vi "CC Script GUI.vi"(10 "Standalone":bool=TRUE, 11 "Cmd Qs":T1) -> ()   [LabVIEW 2024]
uses:
  Subsystems/SS cluster Command Queues.ctl
  Subsystems/SS typedef Cmd Queue Reference.ctl
  Subsystems/SS typedef cluster Instrument Command Queue Data.ctl
  CC cluster Script Panel Defaults.ctl
  typedefs/CC Script Step.ctl
  typedefs/CC enum Script Action.ctl
  typedefs/CC cluster Exposure.ctl
  Detector/Detector Class/Detector enum Detector Integration Mode.ctl
  typedefs/CC cluster Object.ctl
  typedefs/CC cluster sidereal rate.ctl
  typedefs/CC cluster RA and DEC.ctl
  typedefs/cc cluster muRA muDEC.ctl
  Telescope/CC cluster Telescope Offsets.ctl
  Telescope/Telescope cluster Equinox.ctl
  Telescope/Telescope cluster Parallax.ctl
  Telescope/Telescope cluster Rotator.ctl
  Telescope/Telesope ring Frame.ctl
  typedefs/CC cluster Acquire Parameters.ctl
  Subsystems/SS cluster Script Status Queue.ctl
  typedefs/CC cluster Random Dithering.ctl
  typedefs/CC Dithering.ctl
  typedefs/CC cluster Offset Dithering.ctl
  typedefs/CC Dithering Offsets.ctl
  typedefs/CC cluster Observation Record.ctl
  Subsystems/SS cluster New Image Data.ctl
  Subsystems/SS cluster Data Queue type.ctl
  typedefs/CC cluster Observation.ctl
  Observation Queue/CC enum Observation Status.ctl
  typedefs/CC cluster Observation Dither Options.ctl
  typedefs/CC enum Dither Selection.ctl
  hk-channel-class/hk-channel-class/HK Item/HK Item.lvclass
  typedefs/CC cluster Script.ctl
  typedefs/CC cluster Script Status Data.ctl
  typedefs/CC cluster Pause Parameters.ctl
  Filter Wheel/FW cmd Q Move Parameters.ctl
  Logging/CC enum Current Values Action.ctl
  Focus/Focus cluster MoveFocus Command Parameters.ctl
  typedefs/CC cluster Outlet Control.ctl
  CC Rd Wr Script Action.ctl
  e34a80dd-ae96-40f3-85ec-da568b1fc0c6.vi
  a150fa46-afdd-46f6-953a-6d695ab3cc3f.vi
  fb980131-14b8-4ba4-a5ba-d8795c8df878.vi
  73e8f019-b90d-454d-a375-f578a22e9470.vi
  6180e3d0-9506-4a5f-afbf-da5a1e2ce68c.vi
  79eba822-2b6b-4a1a-8f0f-f154aabb2b36.vi
  hk-channel-class/hk-channel-class/HK Table/HK Table.lvclass
  <vilib>/Utility/Data Type/NI_Data Type.lvlib
panel:
  in  "Script Path":path
  in  "Pause Button":bool
  out "Running":bool
  in  "Close":bool
  in  "Stop Script":bool
  in  "New Script":bool
  in  "Edit Script":bool
  in  "Run Script":bool
  in  "Script":string(combo)
  in  "Script":i32(listbox)
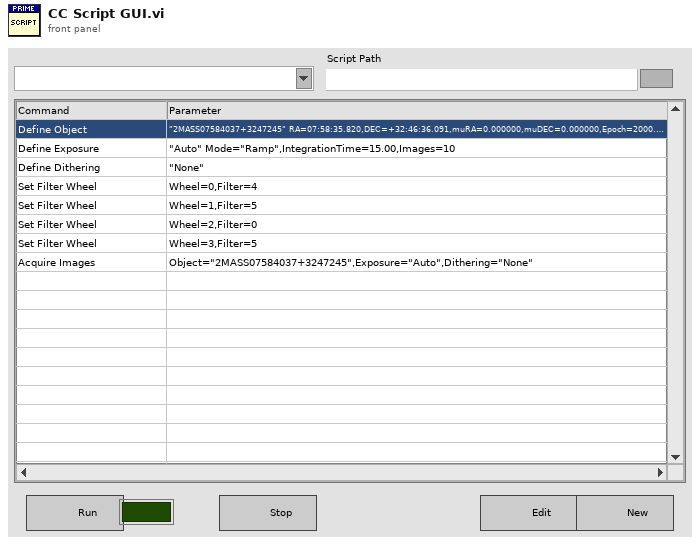
[diagram p1: front panel]
types:
  T1 = typedef "SS cluster Command Queues.ctl" = cluster{"Telescope Q":T2, "Filter Wheel Q":T2, "Script Q":T2, "CryoServer Q":T2, "Detector Q":T2, "Focus Q":T2, "Temp Ctl 1":T2, "Temp Ctl 2":T2, "Temp Ctl 3":T2, "CryoCooler Q":T2, "Pressure Q":T2}
  T2 = typedef "SS typedef Cmd Queue Reference.ctl" = refnum<queue>
  T3 = typedef "CC cluster Telescope Offsets.ctl" = cluster{"xi":dbl, "eta":dbl, "Offset Type":enum16{"SIMPLE", "TPLANE", "PA"}}
  T4 = typedef "CC cluster Script Panel Defaults.ctl" = cluster{"Script Name":string, "Script Path":path}
  T5 = typedef "CC Script Step.ctl" = cluster{"Action":T6, "Data":variant}
  T6 = typedef "CC enum Script Action.ctl" = enum16{"Noop", "Define Object", "Define Exposure", "Define Dithering", "Acquire Images", "Set Filter Wheel", "Telescope Home", "Telescope Move", "Telescope RA DEC", "Focus Move Relative", "Focus Move Absolute", "Focus Set Home", "Macro", "Pause", "Ask User", "Define Random Dither", "CmdLine", "Outlet"}
  T7 = typedef "CC cluster Exposure.ctl" = cluster{"Mode":T8, "Integration Time":dbl, "Name":string, "Images":i32}
  T8 = typedef "Detector enum Detector Integration Mode.ctl" = enum16{"Ramp", "CDS", "FOWLER2", "FOWLER4", "FOWLER8", "FOWLER16", "Raw"}
  T9 = typedef "CC cluster Object.ctl" = cluster{"Object":cluster{"Name":string}, "Sidereal Rate":T10, "RA and DEC":T11, "Proper Motion":T12, "Offsets":T3, "Equinox":T13, "Parallax":T14, "Rotator":T15, "Frame":T16, "Frac Rate":dbl, "Wavelength":dbl}
  T10 = typedef "CC cluster sidereal rate.ctl" = cluster{"dRA":dbl, "dDEC":dbl}
  T11 = typedef "CC cluster RA and DEC.ctl" = cluster{"RA":dbl, "DEC":dbl}
  T12 = typedef "cc cluster muRA muDEC.ctl" = cluster{"muRA":dbl, "muDEC":dbl, "Epoch":dbl}
  T13 = typedef "Telescope cluster Equinox.ctl" = cluster{"Equinox Year":i32, "Equinox Prefix":string}
  T14 = typedef "Telescope cluster Parallax.ctl" = cluster{"Parallax":dbl, "rv kps":dbl}
  T15 = typedef "Telescope cluster Rotator.ctl" = cluster{"Frame":enum16{"Target", "Fixed"}, "PA":dbl}
  T16 = typedef "Telesope ring Frame.ctl" = enum16{"FK4", "FK5", "APPT", "GAPPT", "AZEL"}
  T17 = typedef "CC cluster Acquire Parameters.ctl" = cluster{"Object":string, "Exposure":string, "Dithering":string}
  T18 = typedef "CC cluster Random Dithering.ctl" = cluster{"Count":i32, "Radius":dbl, "Name":string}
  T19 = typedef "CC Dithering.ctl" = cluster{"Name":string, "Dithering Offsets":T20}
  T20 = typedef "CC cluster Offset Dithering.ctl" = cluster{"Offsets":T21[]}
  T21 = typedef "CC Dithering Offsets.ctl" = cluster{"DEC":dbl, "RA":dbl}
  T22 = typedef "CC cluster Observation Record.ctl" = cluster{"Start Time":timestamp, "Script":string, "Object":string, "Detector Settings":string, "Dithering Type":string, "Filter":string, "Images":i32}
  T23 = typedef "SS cluster New Image Data.ctl" = cluster{"Frame number":i32, "Detector #":u16, "FITS file":path, "File size":i64, "Image Type":string}
  T24 = typedef "CC cluster Observation.ctl" = cluster{"Priority":i32, "ID":string, "Observer":string, "Obj Name":string, "Obj Type":string, "RA and DEC String":cluster{"RA":string, "DEC":string}, "Filters":string[], "Integration Time":dbl, "Observation Status":T25, "Offsets":T3, "Images":i32, "Dither Options":T26, "Comment 1":string, "Comment 2":string, "Rotator":T15}
  T25 = typedef "CC enum Observation Status.ctl" = enum16{"Ready", "Running", "Done", "Error"}
  T26 = typedef "CC cluster Observation Dither Options.ctl" = cluster{"Dither":T27, "Dither Radius":dbl, "Dither Points":i32, "Dither Phase":dbl, "B Offset":T11}
  T27 = typedef "CC enum Dither Selection.ctl" = enum16{"None", "Circle", "Random", "ABBA", "OnOff"}
  T28 = cluster{"state":refnum<user-event>, "Script Settings":T4, "Script":T5[], "Cmd Qs":T1, "Parameters":variant, "step":i32, "Script Running":bool, "timer":timestamp, "Script State":string, "Exposure":T7, "Object Map":map{string, T9}, "Acq Settings":T17, "target":T9, "Exp Map":map{string, T7}, "Script Status Q":refnum<queue>, "Images Received":bool, "script edit ref":refnum<vi>, "Run Script":T5[], "Dither":cluster{"Dither Type":bool, "Random Dither":T18, "Offset Dithering":T19, "index":i32}, "Obs List":T22[], "Obs":T22, "images":T23[], "Data Q":refnum<queue>, "Total Images":i32, "paused":bool, "Target RA and DEC":T11, "Image idx":i32, "Observation":T24, "Channel List":refnum<class "HK Item.lvclass">[], "Dither Map":map{string, cluster{"Dither Type":bool, "Random Dither":T18, "Offset Dithering":T19, "index":i32}}, "move start":timestamp, "at slit?":bool, "obj name":string}
  T29 = enum8{"Enabled", "Disabled", "Disabled and Grayed Out"}
  T30 = typedef "SS typedef cluster Instrument Command Queue Data.ctl" = cluster{"Cmd":string, "Parameters":variant}
  T31 = typedef "SS cluster Data Queue type.ctl" = cluster{"Source":string, "Type":string, "Data":variant}
  T32 = typedef "SS cluster Script Status Queue.ctl" = cluster{"Msg":string, "Data":variant}
  T33 = typedef "CC cluster Script.ctl" = cluster{"Name":string, "Script":T5[]}
  T34 = cluster{"Dither Type":bool, "Random Dither":T18, "Offset Dithering":T19, "index":i32}
  T35 = typedef "CC cluster Script Status Data.ctl" = cluster{"Time":timestamp, "Running":bool, "Step":i32, "Script Name":string, "Step Name":string}
  T36 = typedef "CC cluster Pause Parameters.ctl" = cluster{"Time (s)":dbl}
  T37 = typedef "CC enum Current Values Action.ctl" = enum16{"Init", "Write Item", "Write Array", "Read Item", "Read Array", "Read All", "Add Channels", "New File", "Add Message", "Get Current Values", "Close"}
  T38 = typedef "FW cmd Q Move Parameters.ctl" = cluster{"Wheel ID":i32, "Position":i32}
  T39 = typedef "Focus cluster MoveFocus Command Parameters.ctl" = cluster{"Motor":i32, "Position":i32}
  T40 = typedef "CC cluster Outlet Control.ctl" = cluster{"Outlet Idx":i32, "State":bool}
  T41 = typedef "CC Rd Wr Script Action.ctl" = enum16{"Read", "Write", "List", "Delete"}
  T42 = map{string, cluster{"Dither Type":bool, "Random Dither":T18, "Offset Dithering":T19, "index":i32}}
  T43 = typedef "CC cluster Dithering.ctl" = cluster{"Dither Type":bool, "Random Dither":T18, "Offset Dithering":T19, "index":i32}
  T44 = typedef "LVPoint32TypeDef.ctl" = cluster{"Horizontal":i32, "Vertical":i32}
  T45 = typedef "LVRowAndColumnTypeDef.ctl" = cluster{"Row":i32, "Column":i32}
  T46 = enum32{"Invalid", "Standard", "Closed", "Hidden", "Minimized", "Maximized"}
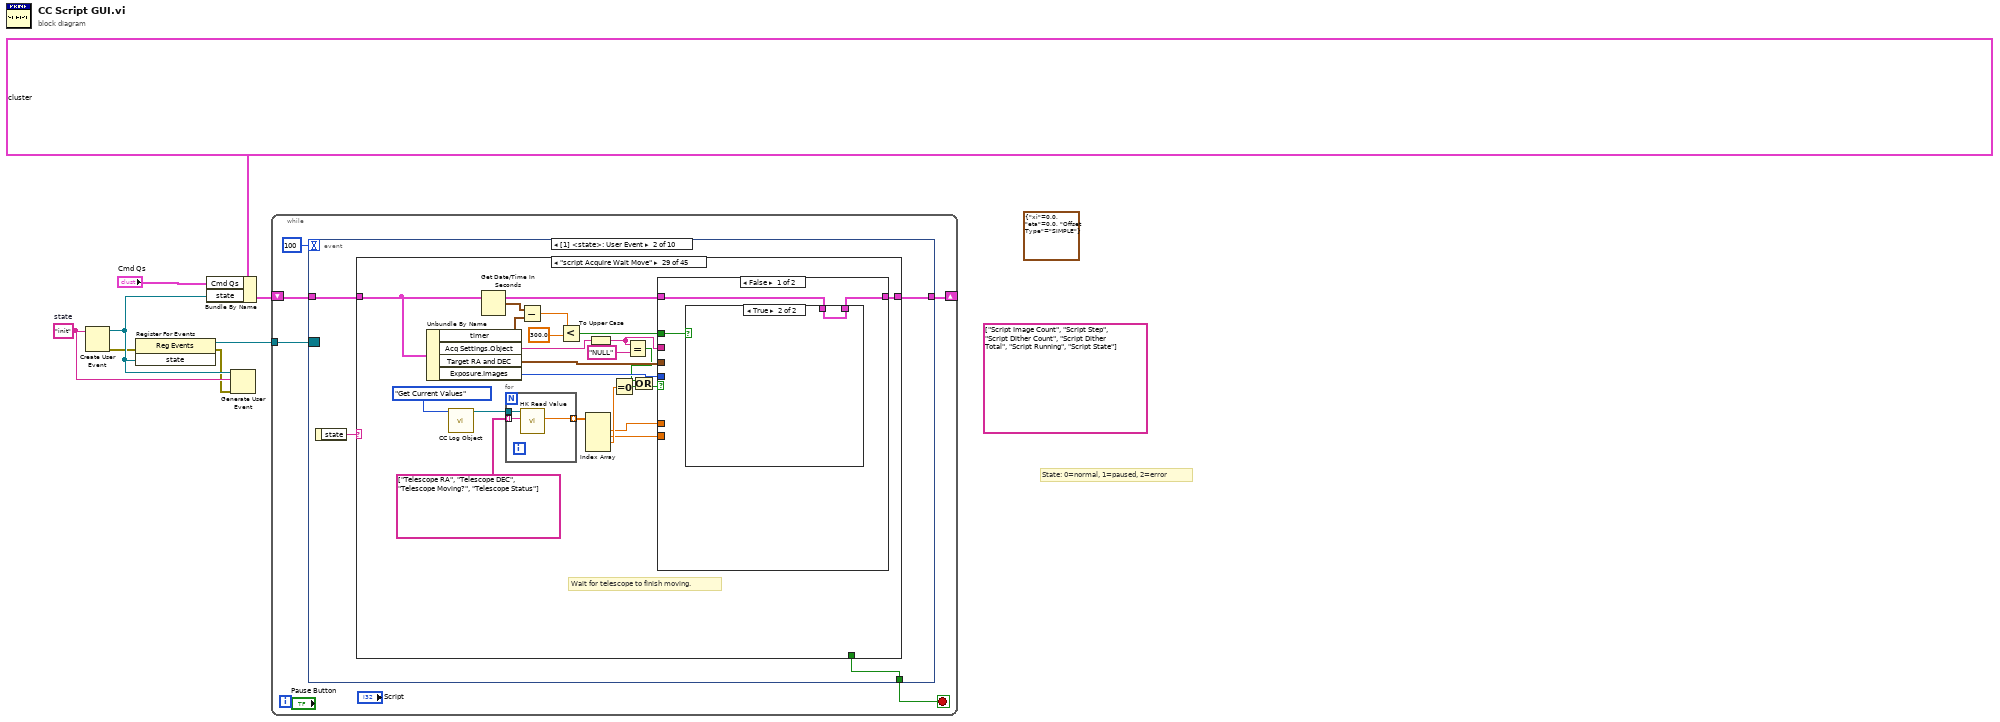
[diagram p0: block diagram]
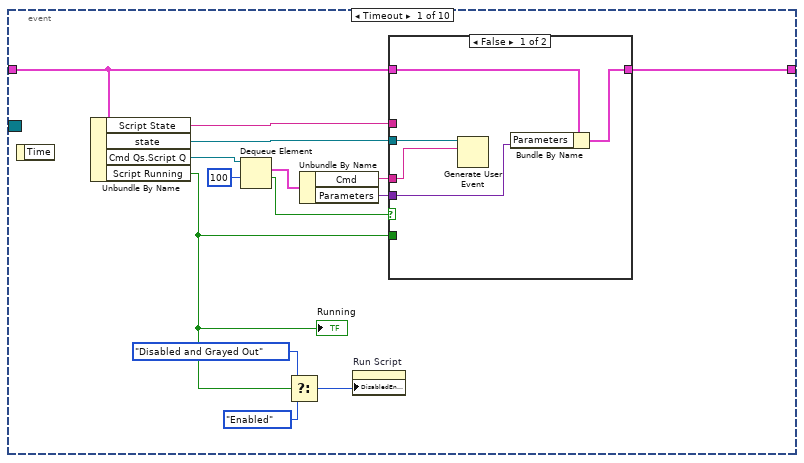
[diagram p2: hidden frame]
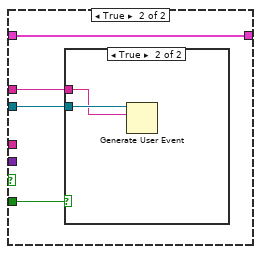
[diagram p3: hidden frame]
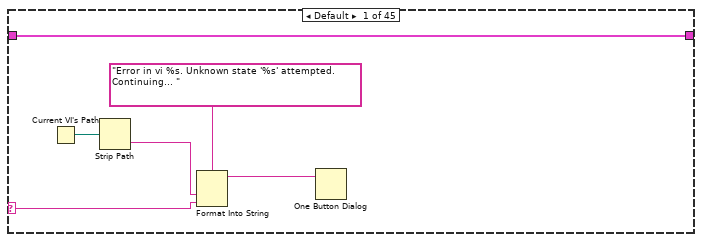
[diagram p5: hidden frame]
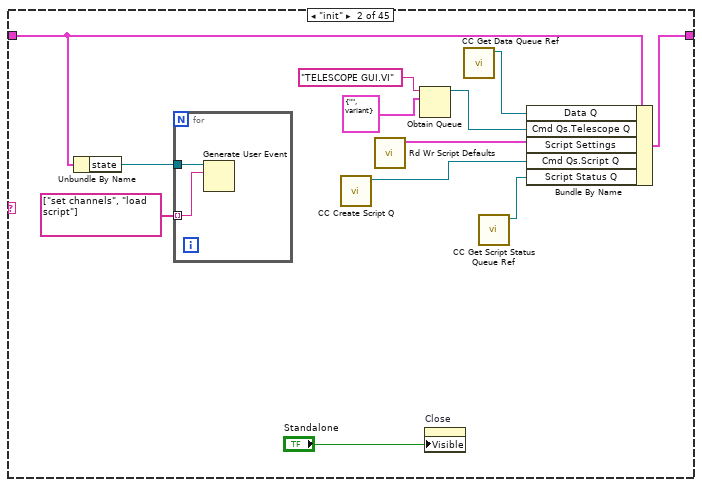
[diagram p6: hidden frame]
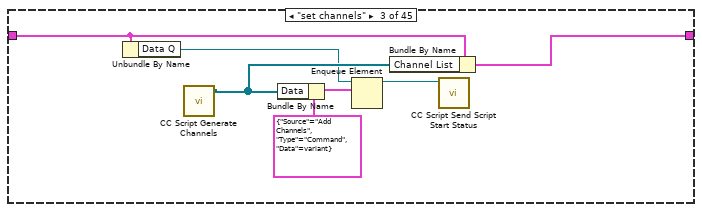
[diagram p7: hidden frame]
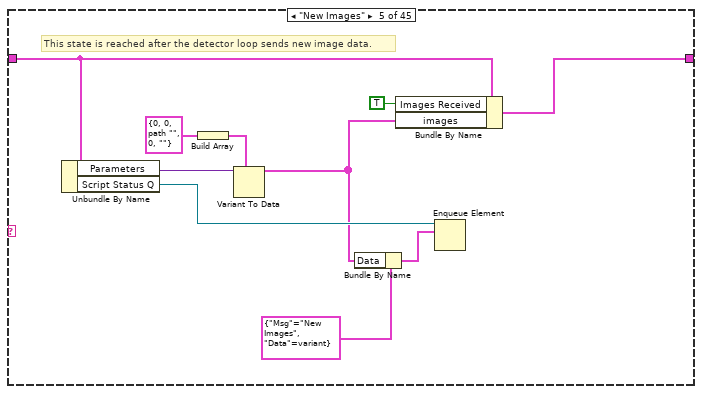
[diagram p9: hidden frame]
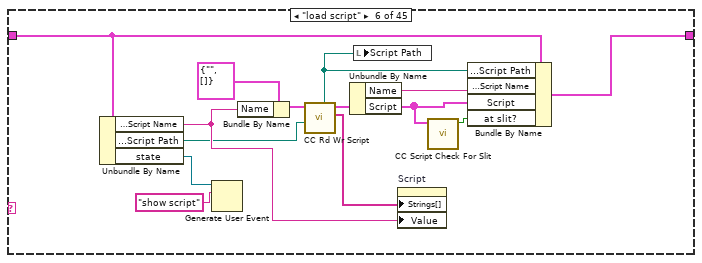
[diagram p10: hidden frame]
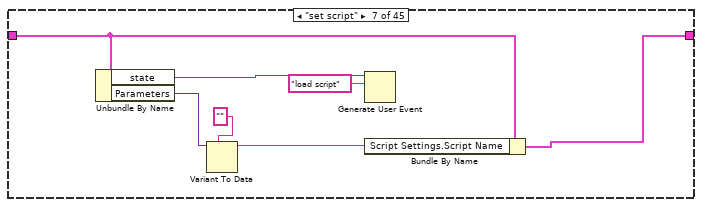
[diagram p11: hidden frame]
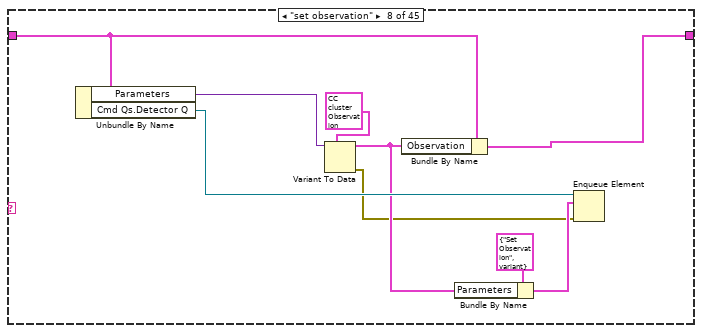
[diagram p12: hidden frame]
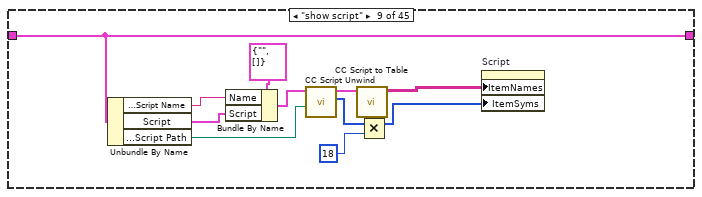
[diagram p13: hidden frame]
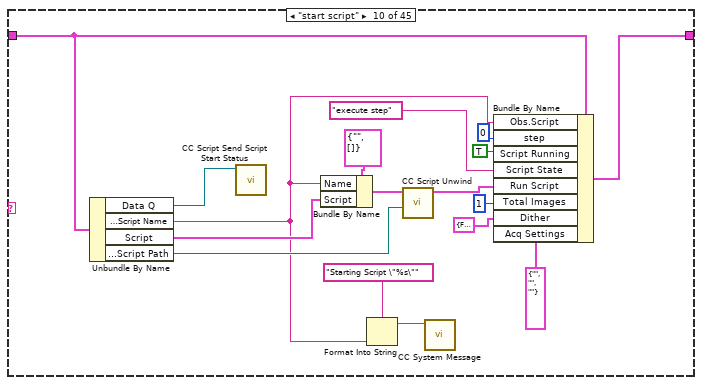
[diagram p14: hidden frame]
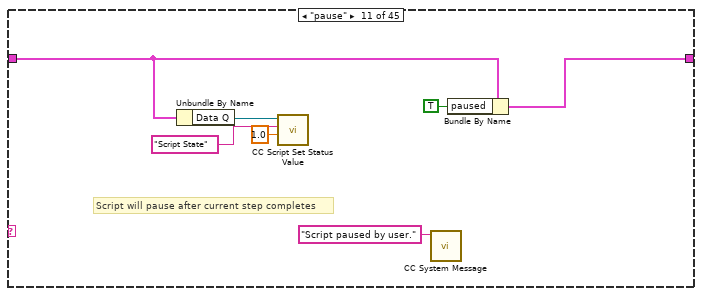
[diagram p15: hidden frame]
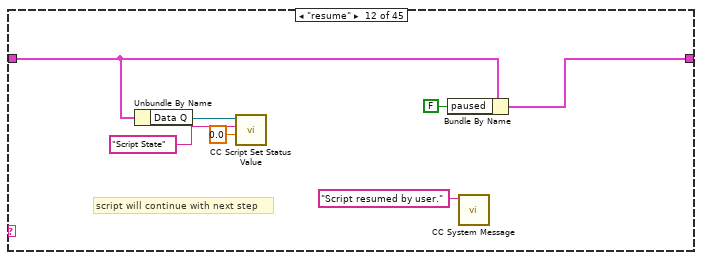
[diagram p16: hidden frame]
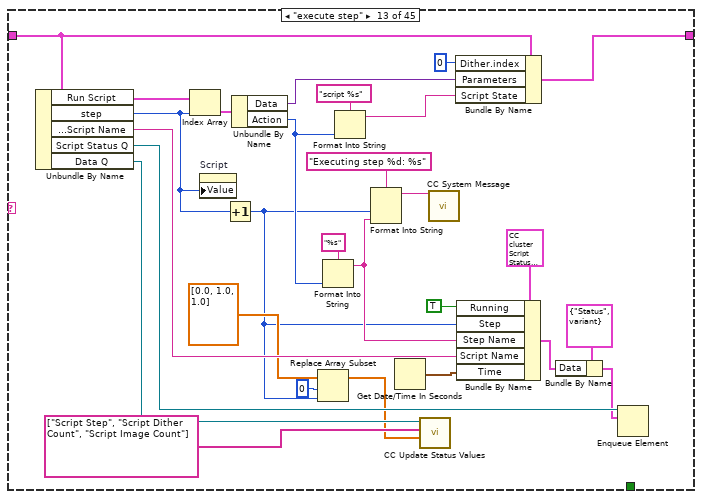
[diagram p17: hidden frame]
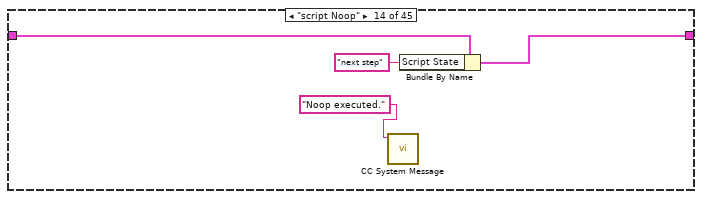
[diagram p18: hidden frame]
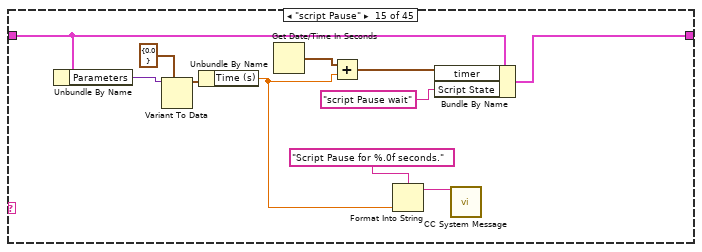
[diagram p19: hidden frame]
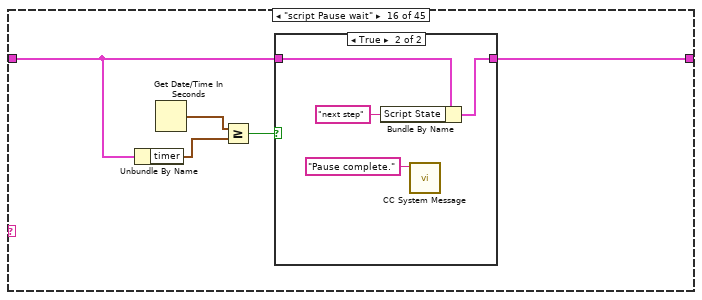
[diagram p20: hidden frame]
diagram:
  (unwired) T3 {"xi"=0.0, "eta"=0.0, "Offset Type"=enum."SIMPLE"} ("Offsets")
  (unwired) string[] ["Script Image Count", "Script Step", "Script Dither Count", "Script Dither Total", "Script Running", "Script State"]
  w4 = "init"  # state
  # "State: 0=normal, 1=paused, 2=error"
  n1 = Create User Event(user event datatype=w4) -> (user event=w6:refnum<user-event>, error out=w2:errorcluster)  [unwired: 1 in]
  n2 = register-events(error in=w2, w6) -> (reference out=w5:refnum<event-registration>, error out=w3:errorcluster)  [unwired: 1 in]
  n3 = Bundle By Name(cluster=T28 {"state"=refnum, "Script Settings"={"Script Name"="", "Script Path"=path ""}, "Script"=[], "Cmd Qs"={"Telescope Q"=refnum, "Filter Wheel Q"=refnum, "Script Q"=refnum, "CryoServer Q"=refnum, "Detector Q"=refnum, "Focus Q"=refnum, "Temp Ctl 1"=refnum, "Temp Ctl 2"=refnum, "Temp Ctl 3"=refnum, "CryoCooler Q"=refnum, "Pressure Q"=refnum}, "Parameters"=variant, "step"=0, "Script Running"=FALSE, "timer"=timestamp(0 s since 1904-01-01), "Script State"="", "Exposure"={"Mode"=enum."CDS", "Integration Time"=1.0, "Name"="", "Images"=1}, "Object Map"={}, "Acq Settings"={"Object"="", "Exposure"="", "Dithering"=""}, "target"={"Object"={"Name"=""}, "Sidereal Rate"={"dRA"=0.0, "dDEC"=0.0}, "RA and DEC"={"RA"=0.0, "DEC"=0.0}, "Proper Motion"={"muRA"=0.0, "muDEC"=0.0, "Epoch"=0.0}, "Offsets"={"xi"=0.0, "eta"=0.0, "Offset Type"=enum."SIMPLE"}, "Equinox"={"Equinox Year"=2000, "Equinox Prefix"="J"}, "Parallax"={"Parallax"=0.0, "rv kps"=0.0}, "Rotator"={"Frame"=enum."Target", "PA"=0.0}, "Frame"=enum."FK5", "Frac Rate"=1.0, "Wavelength"=0.5}, "Exp Map"={}, "Script Status Q"=refnum, "Images Received"=FALSE, "script edit ref"=refnum, "Run Script"=[], "Dither"={"Dither Type"=FALSE, "Random Dither"={"Count"=1, "Radius"=1.0, "Name"=""}, "Offset Dithering"={"Name"="", "Dithering Offsets"={"Offsets"=[]}}, "index"=0}, "Obs List"=[], "Obs"={"Start Time"=timestamp(0 s since 1904-01-01), "Script"="", "Object"="", "Detector Settings"="", "Dithering Type"="", "Filter"="", "Images"=0}, "images"=[], "Data Q"=refnum, "Total Images"=0, "paused"=FALSE, "Target RA and DEC"={"RA"=0.0, "DEC"=0.0}, "Image idx"=0, "Observation"={"Priority"=0, "ID"="", "Observer"="", "Obj Name"="", "Obj Type"="", "RA and DEC String"={"RA"="HH:MM:SS.nnn", "DEC"="DEG:arcmin:arcsec.nn"}, "Filters"=[], "Integration Time"=0.0, "Observation Status"=enum."Ready", "Offsets"={"xi"=0.0, "eta"=0.0, "Offset Type"=enum."SIMPLE"}, "Images"=0, "Dither Options"={"Dither"=enum."None", "Dither Radius"=0.0, "Dither Points"=0, "Dither Phase"=0.0, "B Offset"={"RA"=0.0, "DEC"=0.0}}, "Comment 1"="", "Comment 2"="", "Rotator"={"Frame"=enum."Target", "PA"=0.0}}, "Channel List"=[], "Dither Map"={}, "move start"=timestamp(0 s since 1904-01-01), "at slit?"=FALSE, "obj name"=""}, "Cmd Qs"="Cmd Qs", "state"=w6) -> (w7:T28)
  n4 = Generate User Event(user event=w6, event data cluster=w4, error in=w3) -> ()  [unwired: 1 in, 2 out]
  n5 = while {
    tunnel: w5 -> [w13]
    shift-right: [w11] -> _
    shift-left: w7 -> [w12]
    stop <- w10 stop-if-true
    n6 = event shown="[1] <state>: User Event" {
      selector: w13 -> [_ _ _ _ _ _ _ _ _ _]
      dyn-events: _ -> [_ _ _ _ _ _ _ _ _ _]
      timeout: 100 -> [_ _ _ _ _ _ _ _ _ _]
      tunnel: w12 -> [w21 w41 w755 w758 w773 w815 w820 w842 w845 w848]
      tunnel: [w19 w40 w752 w758 w772 w816 w821 w842 w845 w848] -> w11
      tunnel: [_ w39 _ _ _ _ _ _ _ _] -> w10
      event Timeout {
        n7 = event-data() -> ()  [unwired: 1 in, 1 out]
        n8 = Unbundle By Name(w21) -> ("Script State"=w18:string, "state"=w22:refnum<user-event>, "Cmd Qs.Script Q"=w27:T2, "Script Running"=w17:bool)
        "Running" <- w17
        n9 = Dequeue Element(queue=w27, timeout in ms (-1)=100) -> (element=w25:T30, timed out?=w24:bool)  [unwired: 1 in, 2 out]
        n10 = Select(t=T29."Disabled and Grayed Out" ("Disabled"), s=w17, f=T29."Enabled" ("Disabled")) -> (s? t:f=w14:T29)
        n11 = Unbundle By Name(w25) -> ("Cmd"=w23:string, "Parameters"=w20:variant)
        n12 = property on="Run Script" class="Bool"("DisabledEnum"=w14) -> ()  [unwired: 2 in, 2 out]
        n13 = case shown="False" w24 {
          tunnel: w23 -> [w31 _]
          tunnel: w22 -> [w32 w34]
          tunnel: w21 -> [w30 w36]
          tunnel: w20 -> [w29 _]
          tunnel: [w28 w36] -> w19
          tunnel: w17 -> [_ w35]
          tunnel: w18 -> [_ w33]
          frame False {
            n14 = Generate User Event(user event=w32, event data cluster=w31) -> ()  [unwired: 2 in, 2 out]
            n15 = Bundle By Name(cluster=w30, "Parameters"=w29) -> (w28:T28)
          }
          frame True {
            n16 = case shown="True" w35 {
              tunnel: w34 -> [_ w38]
              tunnel: w33 -> [_ w37]
              frame False {
              }
              frame True {
                n17 = Generate User Event(user event=w38, event data cluster=w37) -> ()  [unwired: 2 in, 2 out]
              }
            }
          }
        }
      }
      event User Event {
        n18 = event-data() -> ("state"=w42:string)  [unwired: 1 in]
        n19 = case shown="\"script Acquire Wait Move\"" w42 {
          selector: w42 -> [w47 _ _ _ _ _ _ _ _ _ _ _ _ _ _ _ _ _ _ _ _ _ w339 _ _ _ w388 _ _ _ w515 _ _ _ _ _ _ _ _ _ _ _ _ _ _]
          tunnel: w41 -> [w43 w58 w65 w70 w75 w86 w96 w108 w121 w137 w140 w150 w172 w181 w186 w197 w210 w242 w261 w281 w301 w332 w341 w364 w374 w385 w390 w426 w450 w498 w512 w527 w552 w576 w589 w612 w626 w650 w651 w666 w693 w721 w729 w740 w748]
          tunnel: [w43 w59 w66 w70 w76 w87 w97 w109 w121 w138 w144 w151 w173 w182 w187 w196 w213 w243 w264 w284 w304 w306 w342 w366 w376 w387 w391 w427 w453 w499 w513 w529 w550 w577 w590 w613 w627 w650 w652 w667 w691 w722 w730 w744 w748] -> w40
          tunnel: [_ _ _ _ _ _ _ _ _ _ _ _ _ _ _ _ _ _ _ _ _ _ _ _ _ _ _ _ _ _ _ _ _ _ _ _ _ _ _ _ _ _ _ _ TRUE] -> w39
          frame Default {
            n20 = Current VI's Path() -> (path=w46:path)
            n21 = Strip Path(path=w46) -> (name=w45:string)  [unwired: 1 out]
            n22 = Format Into String(format string="Error in vi %s. Unknown state '%s' attempted. Continuing... ", w45, w47) -> (resulting string=w44:string)  [unwired: 2 in, 1 out]
            n23 = One Button Dialog(message=w44) -> ()  [unwired: 1 in, 1 out]
          }
          frame "init" {
            n24 = Unbundle By Name(w58) -> ("state"=w57:refnum<user-event>)
            n25 = for {
              tunnel: w57 -> [w62]
              tunnel: string[] ["set channels", "load script"] -> [w61] mode=indexing
              n26 = Generate User Event(user event=w62, event data cluster=w61) -> ()  [unwired: 2 in, 2 out]
            }
            n27 = call "CC Create Script Q.vi"() -> ("Script Q"=w49:refnum<queue>)  [unwired: 10 in, 1 out]
            n28 = call "Rd Wr Script Defaults.vi"() -> ("Script Settings"=w60:T4)  [unwired: 10 in, 1 out]
            n29 = Obtain Queue(name (unnamed)="TELESCOPE GUI.VI", element data type=T30 {"Cmd"="", "Parameters"=variant}) -> (queue out=w52:refnum<queue>)  [unwired: 3 in, 2 out]
            n30 = property on="Close" class="Bool"("Visible"="Standalone") -> ()  [unwired: 2 in, 2 out]
            n31 = call "CC Get Data Queue Ref.vi"() -> ("Data Q"=w50:refnum<queue>)  [unwired: 10 in, 1 out]
            n32 = call "CC Get Script Status Queue Ref.vi"() -> ("Script Status Q"=w55:refnum<queue>)  [unwired: 10 in, 1 out]
            n33 = Bundle By Name(cluster=w58, "Data Q"=w50, "Cmd Qs.Telescope Q"=w52, "Script Settings"=w60, "Cmd Qs.Script Q"=w49, "Script Status Q"=w55) -> (w59:T28)
          }
          frame "set channels" {
            n34 = Unbundle By Name(w65) -> ("Data Q"=w64:refnum<queue>)
            n35 = call "CC Script Generate Channels.vi"() -> ("Channel List"=w67:refnum<class "HK Item.lvclass">[])  [unwired: 9 in, 2 out]
            n36 = Bundle By Name(cluster=T31 {"Source"="Add Channels", "Type"="Command", "Data"=variant} ("element"), "Data"=w67) -> (w69:T31)
            n37 = Enqueue Element(queue=w64, element=w69) -> (queue out=w63:refnum<queue>)  [unwired: 2 in, 2 out]
            n38 = Bundle By Name(cluster=w65, "Channel List"=w67) -> (w66:T28)
            n39 = call "CC Script Send Script Start Status.vi"("Data Q"=w63) -> ()  [unwired: 10 in, 1 out]
          }
          frame "idle" {
          }
          frame "New Images" {
            # "This state is reached after the detector loop sends new image data."
            n40 = Unbundle By Name(w75) -> ("Parameters"=w79:variant, "Script Status Q"=w74:refnum<queue>)
            n41 = Build Array(T23 {"Frame number"=0, "Detector #"=0, "FITS file"=path "", "File size"=0, "Image Type"=""} ("New Image")) -> (w78:T23[])
            n42 = Variant To Data(type=w78, Variant=w79) -> (data=w71:T23[])  [unwired: 1 in, 1 out]
            n43 = Bundle By Name(cluster=T32 {"Msg"="New Images", "Data"=variant} ("element"), "Data"=w71) -> (w72:T32)
            n44 = Bundle By Name(cluster=w75, "Images Received"=TRUE, "images"=w71) -> (w76:T28)
            n45 = Enqueue Element(queue=w74, element=w72) -> ()  [unwired: 2 in, 3 out]
          }
          frame "load script" {
            n46 = Unbundle By Name(w86) -> ("Script Settings.Script Name"=w85:string, "Script Settings.Script Path"=w84:path, "state"=w89:refnum<user-event>)
            n47 = Generate User Event(user event=w89, event data cluster="show script" ("event data")) -> ()  [unwired: 2 in, 2 out]
            n48 = Bundle By Name(cluster=T33 {"Name"="", "Script"=[]} ("Script"), "Name"=w85) -> (w94:T33)
            n49 = call "CC Rd Wr Script.vi"("Script Path"=w84, "Script"=w94) -> ("Script List"=w92:string[], "Script"=w93:T33, "Script Path"=w83:path)  [unwired: 4 in, 3 out]
            n50 = Unbundle By Name(w93) -> ("Name"=w88:string, "Script"=w82:T5[])
            n51 = local write "Script Path"(w83) -> ()
            n52 = property on="Script" class="CmbBox"("Strings[]"=w92, "Value"=w85) -> ()  [unwired: 2 in, 2 out]
            n53 = call "CC Script Check For Slit.vi"("Script"=w82) -> ("At Slit?"=w81:bool)  [unwired: 9 in, 1 out]
            n54 = Bundle By Name(cluster=w86, "Script Settings.Script Path"=w83, "Script Settings.Script Name"=w88, "Script"=w82, "at slit?"=w81) -> (w87:T28)
          }
          frame "set script" {
            n55 = Unbundle By Name(w96) -> ("state"=w99:refnum<user-event>, "Parameters"=w101:variant)
            n56 = Variant To Data(type="", Variant=w101) -> (data=w98:string)  [unwired: 1 in, 1 out]
            n57 = Generate User Event(user event=w99, event data cluster="load script" ("event data")) -> ()  [unwired: 2 in, 2 out]
            n58 = Bundle By Name(cluster=w96, "Script Settings.Script Name"=w98) -> (w97:T28)
          }
          frame "set observation" {
            n59 = Unbundle By Name(w108) -> ("Parameters"=w110:variant, "Cmd Qs.Detector Q"=w106:T2)
            n60 = Variant To Data(type=T24 {"Priority"=0, "ID"="", "Observer"="", "Obj Name"="", "Obj Type"="", "RA and DEC String"={"RA"="HH:MM:SS.nnn", "DEC"="DEG:arcmin:arcsec.nn"}, "Filters"=[], "Integration Time"=0.0, "Observation Status"=enum."Error", "Offsets"={"xi"=0.0, "eta"=0.0, "Offset Type"=enum."SIMPLE"}, "Images"=0, "Dither Options"={"Dither"=enum."None", "Dither Radius"=0.0, "Dither Points"=0, "Dither Phase"=0.0, "B Offset"={"RA"=0.0, "DEC"=0.0}}, "Comment 1"="", "Comment 2"="", "Rotator"={"Frame"=enum."Target", "PA"=0.0}} ("element"), Variant=w110) -> (data=w103:T24, error out=w102:errorcluster)  [unwired: 1 in]
            n61 = Bundle By Name(cluster=w108, "Observation"=w103) -> (w109:T28)
            n62 = Bundle By Name(cluster=T30 {"Cmd"="Set Observation", "Parameters"=variant} ("element"), "Parameters"=w103) -> (w104:T30)
            n63 = Enqueue Element(queue=w106, element=w104, error in (no error)=w102) -> ()  [unwired: 1 in, 3 out]
          }
          frame "show script" {
            n64 = Unbundle By Name(w121) -> ("Script Settings.Script Name"=w118:string, "Script"=w117:T5[], "Script Settings.Script Path"=w111:path)
            n65 = Bundle By Name(cluster=T33 {"Name"="", "Script"=[]} ("Script"), "Name"=w118, "Script"=w117) -> (w116:T33)
            n66 = call "CC Script Unwind.vi"("Script Path"=w111, "Script"=w116) -> ("Indent"=w114:i32[], "Unwound Script"=w115:T5[])  [unwired: 7 in, 1 out]
            n67 = call "CC Script to Table.vi"("Script"=w115) -> ("table"=w120:string[][])  [unwired: 9 in, 1 out]
            n68 = Multiply(x=w114, y=18) -> (x*y=w113:i32[])
            n69 = property on="Script" class="MCListbox (strict)"("ItemNames"=w120, "ItemSyms"=w113) -> ()  [unwired: 2 in, 2 out]
          }
          frame "start script" {
            n70 = Unbundle By Name(w137) -> ("Data Q"=w125:refnum<queue>, "Script Settings.Script Name"=w126:string, "Script"=w130:T5[], "Script Settings.Script Path"=w127:path)
            n71 = call "CC Script Send Script Start Status.vi"("Data Q"=w125) -> ()  [unwired: 10 in, 1 out]
            n72 = Bundle By Name(cluster=T33 {"Name"="", "Script"=[]} ("Script"), "Name"=w126, "Script"=w130) -> (w129:T33)
            n73 = Format Into String(format string="Starting Script \"%s\"" ("Message"), w126) -> (resulting string=w134:string)  [unwired: 2 in, 1 out]
            n74 = call "CC Script Unwind.vi"("Script Path"=w127, "Script"=w129) -> ("Unwound Script"=w128:T5[])  [unwired: 7 in, 2 out]
            n75 = call "CC System Message.vi"("Message"=w134) -> ()  [unwired: 10 in, 1 out]
            n76 = Bundle By Name(cluster=w137, "Obs.Script"=w126, "step"=0, "Script Running"=TRUE, "Script State"="execute step" ("event data"), "Run Script"=w128, "Total Images"=1 ("Image Count"), "Dither"=T34 {"Dither Type"=FALSE, "Random Dither"={"Count"=0, "Radius"=0.0, "Name"=""}, "Offset Dithering"={"Name"="", "Dithering Offsets"={"Offsets"=[]}}, "index"=0}, "Acq Settings"=T17 {"Object"="", "Exposure"="", "Dithering"=""}) -> (w138:T28)
          }
          frame "pause" {
            # "Script will pause after current step completes"
            n77 = Unbundle By Name(w140) -> ("Data Q"=w143:refnum<queue>)
            n78 = call "CC Script Set Status Value.vi"("Value"=1.0, "Ch Name"="Script State", "Data Q"=w143) -> ()  [unwired: 8 in, 1 out]
            n79 = call "CC System Message.vi"("Message"="Script paused by user.") -> ()  [unwired: 10 in, 1 out]
            n80 = Bundle By Name(cluster=w140, "paused"=TRUE) -> (w144:T28)
          }
          frame "resume" {
            # "script will continue with next step"
            n81 = Unbundle By Name(w150) -> ("Data Q"=w149:refnum<queue>)
            n82 = call "CC Script Set Status Value.vi"("Value"=0.0, "Ch Name"="Script State", "Data Q"=w149) -> ()  [unwired: 8 in, 1 out]
            n83 = Bundle By Name(cluster=w150, "paused"=FALSE) -> (w151:T28)
            n84 = call "CC System Message.vi"("Message"="Script resumed by user.") -> ()  [unwired: 10 in, 1 out]
          }
          frame "execute step" {
            n85 = Unbundle By Name(w172) -> ("Run Script"=w180:T5[], "step"=w176:i32, "Script Settings.Script Name"=w165:string, "Script Status Q"=w163:refnum<queue>, "Data Q"=w158:refnum<queue>)
            n86 = Index Array(array=w180, index=w176) -> (element=w179:T5)
            n87 = property on="Script" class="MCListbox (strict)"("Value"=w176) -> ()  [unwired: 2 in, 2 out]
            n88 = Increment(x=w176) -> (x+1=w154:i32)
            n89 = Unbundle By Name(w179) -> ("Data"=w171:variant, "Action"=w167:T6)
            n90 = Replace Array Subset(array=dbl[] [0.0, 1.0, 1.0] ("Values"), new element=w154, index=0) -> (w153:dbl[])
            n91 = Format Into String(format string="%s", w167) -> (resulting string=w166:string)  [unwired: 2 in, 1 out]
            n92 = Format Into String(format string="script %s", w167) -> (resulting string=w174:string)  [unwired: 2 in, 1 out]
            n93 = Format Into String(format string="Executing step %d: %s", w154, w166) -> (resulting string=w175:string)  [unwired: 2 in, 1 out]
            n94 = Get Date/Time In Seconds() -> (seconds since 1Jan1904=w164:timestamp)
            n95 = call "CC Update Status Values.vi"("Values"=w153, "names"=string[] ["Script Step", "Script Dither Count", "Script Image Count"], "Data Q"=w158) -> ()  [unwired: 8 in, 1 out]
            n96 = call "CC System Message.vi"("Message"=w175) -> ()  [unwired: 10 in, 1 out]
            n97 = Bundle By Name(cluster=w172, "Dither.index"=0, "Parameters"=w171, "Script State"=w174) -> (w173:T28)
            n98 = Bundle By Name(cluster=T35 {"Time"=timestamp(0 s since 1904-01-01), "Running"=FALSE, "Step"=0, "Script Name"="", "Step Name"=""}, "Running"=TRUE, "Step"=w154, "Step Name"=w166, "Script Name"=w165, "Time"=w164) -> (w161:T35)
            n99 = Bundle By Name(cluster=T32 {"Msg"="Status", "Data"=variant} ("element"), "Data"=w161) -> (w160:T32)
            n100 = Enqueue Element(queue=w163, element=w160) -> ()  [unwired: 2 in, 3 out]
          }
          frame "script Noop" {
            n101 = call "CC System Message.vi"("Message"="Noop executed." ("format string")) -> ()  [unwired: 10 in, 1 out]
            n102 = Bundle By Name(cluster=w181, "Script State"="next step" ("event data")) -> (w182:T28)
          }
          frame "script Pause" {
            n103 = Unbundle By Name(w186) -> ("Parameters"=w193:variant)
            n104 = Variant To Data(type=T36 {"Time (s)"=0.0} ("Pause Parameters"), Variant=w193) -> (data=w191:T36)  [unwired: 1 in, 1 out]
            n105 = Unbundle By Name(w191) -> ("Time (s)"=w189:dbl)
            n106 = Get Date/Time In Seconds() -> (seconds since 1Jan1904=w190:timestamp)
            n107 = Add(x=w190, y=w189) -> (x+y=w188:timestamp)
            n108 = Format Into String(format string="Script Pause for %.0f seconds.", w189) -> (resulting string=w194:string)  [unwired: 2 in, 1 out]
            n109 = Bundle By Name(cluster=w186, "timer"=w188, "Script State"="script Pause wait" ("event data")) -> (w187:T28)
            n110 = call "CC System Message.vi"("Message"=w194) -> ()  [unwired: 10 in, 1 out]
          }
          frame "script Pause wait" {
            n111 = Unbundle By Name(w197) -> ("timer"=w199:timestamp)
            n112 = Get Date/Time In Seconds() -> (seconds since 1Jan1904=w200:timestamp)
            n113 = Greater Or Equal?(x=w200, y=w199) -> (x >= y?=w198:bool)
            n114 = case shown="True" w198 {
              tunnel: w197 -> [w201 w205]
              tunnel: [w201 w203] -> w196
              frame False {
              }
              frame True {
                n115 = Bundle By Name(cluster=w205, "Script State"="next step") -> (w203:T28)
                n116 = call "CC System Message.vi"("Message"="Pause complete.") -> ()  [unwired: 10 in, 1 out]
              }
            }
          }
          frame "script Macro" {
            n117 = Unbundle By Name(w210) -> ("Parameters"=w211:variant)
            n118 = Variant To Data(type="", Variant=w211) -> (data=w207:string)  [unwired: 1 in, 1 out]
            n119 = Format Into String(format string="Executing Macro %s" ("Message"), w207) -> (resulting string=w206:string)  [unwired: 2 in, 1 out]
            n120 = Bundle By Name(cluster=w210, "Script State"="next step") -> (w213:T28)
            n121 = call "CC System Message.vi"("Message"=w206) -> ()  [unwired: 10 in, 1 out]
          }
          frame "script Define Object" {
            n122 = Unbundle By Name(w242) -> ("Parameters"=w241:variant, "Object Map"=w239:map{string, T9}, "at slit?"=w219:bool, "Cmd Qs.Telescope Q"=w230:T2)
            n123 = Variant To Data(type=T9 {"Object"={"Name"=""}, "Sidereal Rate"={"dRA"=0.0, "dDEC"=0.0}, "RA and DEC"={"RA"=0.0, "DEC"=0.0}, "Proper Motion"={"muRA"=0.0, "muDEC"=0.0, "Epoch"=0.0}, "Offsets"={"xi"=0.0, "eta"=0.0, "Offset Type"=enum."SIMPLE"}, "Equinox"={"Equinox Year"=2000, "Equinox Prefix"="J"}, "Parallax"={"Parallax"=0.0, "rv kps"=0.0}, "Rotator"={"Frame"=enum."Target", "PA"=0.0}, "Frame"=enum."FK5", "Frac Rate"=1.0, "Wavelength"=0.5} ("Object"), Variant=w241) -> (data=w218:T9)  [unwired: 1 in, 1 out]
            n124 = Unbundle By Name(w218) -> ("Offsets"=w217:T3)
            n125 = Unbundle By Name(w218) -> ("Object.Name"=w229:string)
            n126 = To Variant(anything=w217) -> (Variant=w216:variant)
            n127 = Unbundle By Name(w218) -> ("Object.Name"=w236:string, "RA and DEC.RA"=w235:dbl, "RA and DEC.DEC"=w234:dbl, "Offsets.xi"=w233:dbl, "Offsets.eta"=w232:dbl, "Rotator.PA"=w231:dbl)
            n128 = To Variant(anything=w218) -> (Variant=w215:variant)
            n129 = Get Date/Time In Seconds() -> (seconds since 1Jan1904=w224:timestamp)
            n130 = To Upper Case(1:w229) -> (0:w222:string)
            n131 = Insert Into Map(map in=w239, key=w229, value=w218) -> (map out=w238:map{string, T9})  [unwired: 2 out]
            n132 = Select(t=w216, s=w219, f=w215) -> (s? t:f=w214:variant)
            n133 = Bundle By Name(cluster=w242, "move start"=w224, "Script State"="next step", "obj name"=w222, "Object Map"=w238) -> (w243:T28)
            n134 = Empty String/Path?(string/path=w222) -> (empty?=w220:bool)
            n135 = Equal?(x="NULL" ("y"), y=w222) -> (x = y?=w228:bool)
            n136 = Or(x=w228, y=w220) -> (x .or. y?=w221:bool)
            n137 = Format Into String(format string="Script defined target object \"%s\" at RA=%f, DEC=%f and xi=%.1f, eta=%.1f, ROTPA=%.1g", w236, w235, w234, w233, w232, w231) -> (resulting string=w227:string)  [unwired: 2 in, 1 out]
            n138 = case shown="True" w221 {
              tunnel: w230 -> [w250 _]
              tunnel: w214 -> [w249 _]
              tunnel: w219 -> [w248 _]
              frame False {
                # "Move telescope"
                n139 = Select(t=T30 {"Cmd"="Offset", "Parameters"=variant} ("element"), s=w248, f=T30 {"Cmd"="Move", "Parameters"=variant} ("element")) -> (s? t:f=w245:T30)
                n140 = Bundle By Name(cluster=w245, "Parameters"=w249) -> (w251:T30)
                n141 = Enqueue Element(queue=w250, element=w251) -> ()  [unwired: 2 in, 3 out]
              }
              frame True {
              }
            }
            n142 = Select(t="Script not moving telescope (Null object selected)", s=w221, f=w227) -> (s? t:f=w226:string)
            n143 = call "CC System Message.vi"("Message"=w226) -> ()  [unwired: 10 in, 1 out]
          }
          frame "script Define Exposure" {
            n144 = Unbundle By Name(w261) -> ("Exp Map"=w260:map{string, T7}, "Parameters"=w263:variant)
            n145 = Variant To Data(type=T7 {"Mode"=enum."CDS", "Integration Time"=1.0, "Name"="", "Images"=1} ("Exposure"), Variant=w263) -> (data=w258:T7)  [unwired: 1 in, 1 out]
            n146 = Unbundle By Name(w258) -> ("Images"=w252:i32, "Name"=w255:string, "Mode"=w254:T8, "Integration Time"=w253:dbl)
            n147 = Insert Into Map(map in=w260, key=w255, value=w258) -> (map out=w259:map{string, T7})  [unwired: 2 out]
            n148 = Bundle By Name(cluster=w261, "Script State"="next step", "Exp Map"=w259, "Image idx"=w252) -> (w264:T28)
            n149 = Format Into String(format string="Script defined exposure settings \"%s\" mode %s, integration time %f, collection %d images.", w255, w254, w253, w252) -> (resulting string=w256:string)  [unwired: 2 in, 1 out]
            n150 = call "CC System Message.vi"("Message"=w256) -> ()  [unwired: 10 in, 1 out]
          }
          frame "script Define Random Dither" {
            n151 = Unbundle By Name(w281) -> ("Parameters"=w283:variant, "Dither Map"=w272:T42, "Data Q"=w276:refnum<queue>)
            n152 = Variant To Data(type=T18 {"Count"=1, "Radius"=1.0, "Name"=""} ("Dithering Offsets"), Variant=w283) -> (data=w267:T18)  [unwired: 1 in, 1 out]
            n153 = Unbundle By Name(w267) -> ("Name"=w266:string)
            n154 = Unbundle By Name(w267) -> ("Name"=w278:string, "Count"=w274:i32, "Radius"=w277:dbl)
            n155 = Bundle By Name(cluster=T34 {"Dither Type"=FALSE, "Random Dither"={"Count"=0, "Radius"=0.0, "Name"=""}, "Offset Dithering"={"Name"="", "Dithering Offsets"={"Offsets"=[]}}, "index"=0} ("value"), "Random Dither"=w267, "Dither Type"=TRUE) -> (w268:T34)
            n156 = Increment(x=w274) -> (x+1=w273:i32)
            n157 = Format Into String(format string="Script defined random dithering \"%s\" at %d spots with radius %f", w278, w274, w277) -> (resulting string=w279:string)  [unwired: 2 in, 1 out]
            n158 = call "CC Script Set Status Value.vi"("Value"=w273, "Ch Name"="Script Dither Total", "Data Q"=w276) -> ()  [unwired: 8 in, 1 out]
            n159 = Insert Into Map(map in=w272, key=w266, value=w268) -> (map out=w269:T42)  [unwired: 2 out]
            n160 = call "CC System Message.vi"("Message"=w279) -> ()  [unwired: 10 in, 1 out]
            n161 = Bundle By Name(cluster=w281, "Script State"="next step", "Dither Map"=w269) -> (w284:T28)
          }
          frame "script Define Dithering" {
            n162 = Unbundle By Name(w301) -> ("Parameters"=w303:variant, "Dither Map"=w288:T42, "Data Q"=w295:refnum<queue>)
            n163 = Variant To Data(type=T19 {"Name"="", "Dithering Offsets"={"Offsets"=[]}} ("Dithering Offsets"), Variant=w303) -> (data=w287:T19)  [unwired: 1 in, 1 out]
            n164 = Unbundle By Name(w287) -> ("Name"=w298:string, "Dithering Offsets.Offsets"=w297:T21[])
            n165 = Unbundle By Name(w287) -> ("Name"=w289:string)
            n166 = Bundle By Name(cluster=T34 {"Dither Type"=FALSE, "Random Dither"={"Count"=0, "Radius"=0.0, "Name"=""}, "Offset Dithering"={"Name"="", "Dithering Offsets"={"Offsets"=[]}}, "index"=0} ("value"), "Offset Dithering"=w287, "Dither Type"=FALSE) -> (w290:T34)
            n167 = Array Size(array=w297) -> (size(s)=w294:i32)
            n168 = Insert Into Map(map in=w288, key=w289, value=w290) -> (map out=w286:T42)  [unwired: 2 out]
            n169 = Format Into String(format string="Script defined dithering \"%s\" containing %d offsets.", w298, w294) -> (resulting string=w299:string)  [unwired: 2 in, 1 out]
            n170 = Increment(x=w294) -> (x+1=w293:i32)
            n171 = Bundle By Name(cluster=w301, "Script State"="next step", "Dither Map"=w286) -> (w304:T28)
            n172 = call "CC System Message.vi"("Message"=w299) -> ()  [unwired: 10 in, 1 out]
            n173 = call "CC Script Set Status Value.vi"("Value"=w293, "Ch Name"="Script Dither Total", "Data Q"=w295) -> ()  [unwired: 8 in, 1 out]
          }
          frame "script Set Filter Wheel" {
            n174 = Unbundle By Name(w332) -> ("Parameters"=w333:variant, "Cmd Qs.Filter Wheel Q"=w331:T2)
            n175 = Variant To Data(type=T38 {"Wheel ID"=0, "Position"=0}, Variant=w333) -> (data=w324:T38, error out=w328:errorcluster)  [unwired: 1 in]
            n176 = call "CC Log Object.vi"("Action"=CC_enum_Current_Values_Action."Get Current Values") -> ("HK Channel out"=w322:refnum<class "HK Table.lvclass">)  [unwired: 8 in, 2 out]
            n177 = Bundle By Name(cluster=T30 {"Cmd"="Move", "Parameters"=variant} ("element"), "Parameters"=w324) -> (w325:T30)
            n178 = Unbundle By Name(w324) -> ("Wheel ID"=w313:i32, "Position"=w311:i32)
            n179 = Enqueue Element(queue=w331, element=w325, error in (no error)=w328) -> ()  [unwired: 1 in, 3 out]
            n180 = Bundle By Name(cluster=w332, "Script State"="script Filter Wheel Wait") -> (w308:T28)
            n181 = Format Into String(format string="Wheel%d Filter", w313) -> (resulting string=w320:string)  [unwired: 2 in, 1 out]
            n182 = Equal?(x=3, y=w313) -> (x = y?=w309:bool)
            n183 = call-dynamic "HK Read Value.vi"("Channel Name"=w320, "HK Channel in"=w322) -> ("error out"=w314:errorcluster, "Value"=w319:dbl)  [unwired: 4 in, 4 out]
            n184 = Not Equal?(x=5, y=w311) -> (x != y?=w307:bool)
            n185 = Equal?(x=w311, y=w319) -> (x = y?=w318:bool)
            n186 = Format Into String(format string="Script moving filter wheel %d to position %d", w313, w311) -> (resulting string=w326:string)  [unwired: 2 in, 1 out]
            n187 = case shown="True" w309 {
              tunnel: w308 -> [w335 w338]
              tunnel: w307 -> [_ w337]
              tunnel: [w335 w336] -> w306
              frame False {
              }
              frame True {
                n188 = Bundle By Name(cluster=w338, "at slit?"=w337) -> (w336:T28)
              }
            }
            n189 = Select(t=u32 0, s=w318, f=u32 10000 ("milliseconds to wait")) -> (s? t:f=w316:u32)
            n190 = call "Stall Data Flow.vim"("value in"=w314, "milliseconds to wait"=w316) -> ()  [unwired: 2 out]
            n191 = call "CC System Message.vi"("Message"=w326) -> ()  [unwired: 10 in, 1 out]
          }
          frame "script Filter Wheel Wait" {
            n192 = call "CC Log Object.vi"("Action"=CC_enum_Current_Values_Action."Get Current Values") -> ("HK Channel out"=w349:refnum<class "HK Table.lvclass">)  [unwired: 8 in, 2 out]
            n193 = for {
              N: 4 -> [_]
              tunnel: w349 -> [w355]
              tunnel: [w354] -> w346 mode=indexing
              tunnel: "Wheel%d Moving" -> [w353]
              i -> [w352]
              n194 = Format Into String(format string=w353, w352) -> (resulting string=w351:string)  [unwired: 2 in, 1 out]
              n195 = call-dynamic "HK Read Value.vi"("Channel Name"=w351, "HK Channel in"=w355) -> ("Value"=w354:dbl)  [unwired: 4 in, 5 out]
            }
            n196 = Equal To 0?(x=w346) -> (x = 0?=w345:bool[])
            n197 = And Array Elements(Boolean array=w345) -> (logical AND=w344:bool)
            n198 = Select(t="next step", s=w344, f=w339) -> (s? t:f=w343:string)
            n199 = Bundle By Name(cluster=w341, "Script State"=w343) -> (w342:T28)
          }
          frame "script Focus Move Relative" {
            # "Wait one second to allow focus to start move."
            n200 = Unbundle By Name(w364) -> ("Parameters"=w365:variant, "Cmd Qs.Focus Q"=w363:T2)
            n201 = Variant To Data(type=T39 {"Motor"=0, "Position"=0} ("Cluster"), Variant=w365) -> (data=w361:T39, error out=w360:errorcluster)  [unwired: 1 in]
            n202 = Bundle By Name(cluster=T30 {"Cmd"="FocusMoveRelative", "Parameters"=variant} ("element"), "Parameters"=w361) -> (w359:T30)
            n203 = Enqueue Element(queue=w363, element=w359, error in (no error)=w360) -> (error out=w357:errorcluster)  [unwired: 1 in, 2 out]
            n204 = Bundle By Name(cluster=w364, "Script State"="script Focus Move Wait") -> (w366:T28)
            n205 = call "Stall Data Flow.vim"("value in"=w357, "milliseconds to wait"=u32 1000) -> ()  [unwired: 2 out]
          }
          frame "script Focus Move Absolute" {
            n206 = Unbundle By Name(w374) -> ("Parameters"=w375:variant, "Cmd Qs.Focus Q"=w373:T2)
            n207 = Variant To Data(type=T39 {"Motor"=0, "Position"=0} ("Cluster"), Variant=w375) -> (data=w371:T39, error out=w370:errorcluster)  [unwired: 1 in]
            n208 = Bundle By Name(cluster=T30 {"Cmd"="FocusMoveAbsolute", "Parameters"=variant} ("element"), "Parameters"=w371) -> (w369:T30)
            n209 = Enqueue Element(queue=w373, element=w369, error in (no error)=w370) -> ()  [unwired: 1 in, 3 out]
            n210 = Bundle By Name(cluster=w374, "Script State"="next step") -> (w376:T28)
          }
          frame "script Focus Set Home" {
            n211 = Unbundle By Name(w385) -> ("Parameters"=w386:variant, "Cmd Qs.Focus Q"=w384:T2)
            n212 = Variant To Data(type=0, Variant=w386) -> (data=w382:i32, error out=w381:errorcluster)  [unwired: 1 in]
            n213 = Bundle By Name(cluster=T30 {"Cmd"="FocusSetHome", "Parameters"=variant} ("element"), "Parameters"=w382) -> (w380:T30)
            n214 = Enqueue Element(queue=w384, element=w380, error in (no error)=w381) -> ()  [unwired: 1 in, 3 out]
            n215 = Bundle By Name(cluster=w385, "Script State"="script Focus Move Wait") -> (w387:T28)
          }
          frame "script Focus Move Wait" {
            n216 = call "CC Log Object.vi"("Action"=CC_enum_Current_Values_Action."Get Current Values") -> ("HK Channel out"=w398:refnum<class "HK Table.lvclass">)  [unwired: 8 in, 2 out]
            n217 = for {
              N: 2 -> [_]
              tunnel: w398 -> [w404]
              tunnel: [w403] -> w395 mode=indexing
              tunnel: "Focus Motor %d Moving" -> [w402]
              i -> [w401]
              n218 = Format Into String(format string=w402, w401) -> (resulting string=w400:string)  [unwired: 2 in, 1 out]
              n219 = call-dynamic "HK Read Value.vi"("Channel Name"=w400, "HK Channel in"=w404) -> ("Value"=w403:dbl)  [unwired: 4 in, 5 out]
            }
            n220 = Equal To 0?(x=w395) -> (x = 0?=w394:bool[])
            n221 = And Array Elements(Boolean array=w394) -> (logical AND=w393:bool)
            n222 = Select(t="next step", s=w393, f=w388) -> (s? t:f=w392:string)
            n223 = Bundle By Name(cluster=w390, "Script State"=w392) -> (w391:T28)
          }
          frame "script Acquire Images" {
            # "Telescope move command\nnow in the Define Object\nstep to save time."
            # "Tell the telescope to move to target."
            n224 = Unbundle By Name(w426) -> ("Dither Map"=w407:T42, "Exp Map"=w410:map{string, T7}, "Object Map"=w425:map{string, T9}, "Parameters"=w429:variant, "Data Q"=w416:refnum<queue>)
            n225 = Variant To Data(type=T17 {"Object"="", "Exposure"="", "Dithering"=""} ("Acquire Parameters"), Variant=w429) -> (data=w411:T17)  [unwired: 1 in, 1 out]
            n226 = Unbundle By Name(w411) -> ("Dithering"=w406:string, "Exposure"=w409:string)
            n227 = Unbundle By Name(w411) -> ("Object"=w417:string)
            n228 = call "CC Script Set Status Value.vi"("Value"=1.0, "Ch Name"="Script Dither Count", "Data Q"=w416) -> ()  [unwired: 8 in, 1 out]
            n229 = Remove From Map(10:w417, 11:w425) -> (1:w424:T9, 2:w423:bool)  [unwired: 1 out]
            n230 = Remove From Map(10:w406, 11:w407) -> (1:w405:T34)  [unwired: 2 out]
            n231 = Remove From Map(10:w409, 11:w410) -> (1:w408:T7)  [unwired: 2 out]
            n232 = case shown="False" w423 {
              tunnel: w424 -> [w430 w432]
              tunnel: ["script Acquire Wait Move" ("Script State") "abort script" ("Script State")] -> w422
              tunnel: w417 -> [_ w434]
              tunnel: [w430 w432] -> w413
              frame False {
              }
              frame True {
                n233 = Format Into String(format string="Acquire Images command referred to undefined object \"%s\".", w434) -> (resulting string=w433:string)  [unwired: 2 in, 1 out]
                n234 = call "CC System Message.vi"("Message"=w433) -> ()  [unwired: 10 in, 1 out]
                n235 = One Button Dialog(message=w433) -> ()  [unwired: 1 in, 1 out]
              }
            }
            n236 = Format Into String(format string="Waiting for telescope to target %s", w417) -> (resulting string=w418:string)  [unwired: 2 in, 1 out]
            n237 = Unbundle By Name(w413) -> ("RA and DEC"=w412:T11)
            n238 = call "CC System Message.vi"("Message"=w418) -> ()  [unwired: 10 in, 1 out]
            n239 = Get Date/Time In Seconds() -> (seconds since 1Jan1904=w421:timestamp)
            n240 = Bundle By Name(cluster=w426, "Dither.index"=0, "Acq Settings"=w411, "timer"=w421, "Dither"=w405, "Exposure"=w408, "target"=w413, "Target RA and DEC"=w412, "Script State"=w422) -> (w427:T28)
          }
          frame "script Acquire Wait Move" {
            # "Wait for telescope to finish moving."
            n241 = Unbundle By Name(w450) -> ("timer"=w445:timestamp, "Acq Settings.Object"=w440:string, "Target RA and DEC"=w449:T11, "Exposure.Images"=w442:i32)
            n242 = call "CC Log Object.vi"("Action"=CC_enum_Current_Values_Action."Get Current Values") -> ("HK Channel out"=w457:refnum<class "HK Table.lvclass">)  [unwired: 8 in, 2 out]
            n243 = Get Date/Time In Seconds() -> (seconds since 1Jan1904=w447:timestamp)
            n244 = for {
              tunnel: w457 -> [w461]
              tunnel: string[] ["Telescope RA", "Telescope DEC", "Telescope Moving?", "Telescope Status"] -> [w460] mode=indexing
              tunnel: [w459] -> w455 mode=indexing
              n245 = call-dynamic "HK Read Value.vi"("Channel Name"=w460, "HK Channel in"=w461) -> ("Value"=w459:dbl)  [unwired: 4 in, 5 out]
            }
            n246 = Subtract(x=w447, y=w445) -> (x-y=w448:dbl)
            n247 = Less?(x=w448, y=300.0) -> (x < y?=w444:bool)
            n248 = Index Array(array=w455) -> (element #1=w452:dbl, element #2=w451:dbl, element #3=w454:dbl)  [unwired: 4 in, 1 out]
            n249 = To Upper Case(1:w440) -> (0:w439:string)
            n250 = Equal To 0?(x=w454) -> (x = 0?=w443:bool)
            n251 = Equal?(x=w439, y="NULL") -> (x = y?=w437:bool)
            n252 = Or(x=w437, y=w443) -> (x .or. y?=w438:bool)
            n253 = case shown="False" w438 {
              tunnel: w450 -> [w462 w477]
              tunnel: [w463 w478] -> w453
              tunnel: w452 -> [_ w481]
              tunnel: w451 -> [_ w480]
              tunnel: w449 -> [_ w482]
              tunnel: w444 -> [w464 _]
              tunnel: w442 -> [_ w475]
              tunnel: w439 -> [_ w470]
              frame False {
                n254 = case shown="True" w464 {
                  tunnel: w462 -> [w467 w469]
                  tunnel: [w466 w469] -> w463
                  frame False {
                    n255 = call "CC System Message.vi"("Message"="Timeout waiting for telescope to reach position.") -> ()  [unwired: 10 in, 1 out]
                    n256 = Bundle By Name(cluster=w467, "Script State"="Script Error") -> (w466:T28)
                  }
                  frame True {
                  }
                }
              }
              frame True {
                # "Not moving"
                n257 = Bundle(cluster=w482, "RA"=w481, "DEC"=w480) -> (w479:T11)
                n258 = call "CC Script Check Telescope is Close Enough.vi"("Target Object"=w470, "Current Pos"=w479, "Target Pos"=w482) -> ("msg"=w471:string, "close enough"=w474:bool)  [unwired: 6 in, 1 out]
                n259 = case shown="True" w474 {
                  tunnel: w475 -> [_ w485]
                  tunnel: w471 -> [w483 _]
                  frame False {
                    n260 = call "CC System Message.vi"("Message"=w483) -> ()  [unwired: 10 in, 1 out]
                  }
                  frame True {
                    n261 = Format Into String(format string="Image 1 of %d.", w485) -> (resulting string=w484:string)  [unwired: 2 in, 1 out]
                    n262 = call "CC System Message.vi"("Message"=w484) -> ()  [unwired: 10 in, 1 out]
                  }
                }
                n263 = Select(t="script Read Detectors", s=w474, f="Script Error" ("Script State")) -> (s? t:f=w476:string)
                n264 = Bundle By Name(cluster=w477, "Script State"=w476) -> (w478:T28)
              }
            }
          }
          frame "script Read Detectors" {
            n265 = Unbundle By Name(w498) -> ("Exp Map"=w505:map{string, T7}, "Acq Settings.Exposure"=w504:string, "Cmd Qs.Detector Q"=w503:T2)
            n266 = Remove From Map(10:w504, 11:w505) -> (1:w489:T7)  [unwired: 2 out]
            n267 = Unbundle By Name(w489) -> ("Images"=w490:i32, "Name"=w493:string, "Mode"=w492:T8, "Integration Time"=w491:dbl)
            n268 = Bundle By Name(cluster=T30 {"Cmd"="Acquire Image", "Parameters"=variant} ("element"), "Parameters"=w489) -> (w501:T30)
            n269 = Enqueue Element(queue=w503, element=w501) -> ()  [unwired: 2 in, 3 out]
            n270 = Get Date/Time In Seconds() -> (seconds since 1Jan1904=w497:timestamp)
            n271 = Format Into String(format string="Detector exposure settings \"%s\" mode %s, integration time %f, collection %d images.", w493, w492, w491, w490) -> (resulting string=w487:string)  [unwired: 2 in, 1 out]
            n272 = Bundle By Name(cluster=w498, "timer"=w497, "Script State"="script Wait for Image", "Images Received"=FALSE) -> (w499:T28)
            n273 = call "CC System Message.vi"("Message"="Commanding Detector to acquire images." ("format string")) -> ("error out"=w488:errorcluster)  [unwired: 10 in]
            n274 = call "CC System Message.vi"("error in (no error)"=w488, "Message"=w487) -> ()  [unwired: 9 in, 1 out]
          }
          frame "script Wait for Image" {
            # "Waiting for detector system to return images via script Q. State \"New Images\" sets the state so we can move on."
            n275 = Unbundle By Name(w512) -> ("Images Received"=w516:bool, "Acq Settings"=w511:T17)
            n276 = Unbundle By Name(w511) -> ("Object"=w508:string, "Exposure"=w507:string, "Dithering"=w506:string)
            n277 = Select(t="Next Image", s=w516, f=w515) -> (s? t:f=w514:string)
            n278 = Bundle By Name(cluster=w512, "Obs.Object"=w508, "Obs.Detector Settings"=w507, "Obs.Dithering Type"=w506) -> (w510:T28)
            n279 = Bundle By Name(cluster=w510, "Script State"=w514) -> (w513:T28)
          }
          frame "Next Image" {
            n280 = Unbundle By Name(w527) -> ("Exposure.Images"=w519:i32, "Image idx"=w524:i32, "Data Q"=w526:refnum<queue>, "Total Images"=w525:i32)
            n281 = Increment(x=w525) -> (x+1=w518:i32)
            n282 = Decrement(x=w524) -> (x-1=w522:i32)
            n283 = call "CC Script Set Status Value.vi"("Value"=w518, "Ch Name"="Script Image Count", "Data Q"=w526) -> ()  [unwired: 8 in, 1 out]
            n284 = Greater Than 0?(x=w522) -> (x > 0?=w523:bool)
            n285 = case shown="False" w523 {
              tunnel: w522 -> [_ w537]
              tunnel: [w531 w537] -> w521
              tunnel: ["Next Dither" "script Read Detectors"] -> w520
              tunnel: w519 -> [w531 w535]
              tunnel: ["Images complete. Going to next dither." w534] -> w517
              frame False {
              }
              frame True {
                n286 = Subtract(x=w535, y=w537) -> (x-y=w536:i32)
                n287 = Increment(x=w536) -> (x+1=w533:i32)
                n288 = Format Into String(format string="Image %d of %d.", w533, w535) -> (resulting string=w534:string)  [unwired: 2 in, 1 out]
              }
            }
            n289 = Bundle By Name(cluster=w527, "Image idx"=w521, "Script State"=w520, "Total Images"=w518) -> (w529:T28)
            n290 = call "CC System Message.vi"("Message"=w517) -> ()  [unwired: 10 in, 1 out]
          }
          frame "Next Dither" {
            # "Updated to send \"Offset\" to telescope instead of move command"
            n291 = Unbundle By Name(w552) -> ("Dither"=w548:T34, "target"=w540:T9, "Cmd Qs.Telescope Q"=w553:T2, "Data Q"=w545:refnum<queue>)
            n292 = call "CC Script Next Dither.vi"("object"=w540, "Dither"=w548) -> ("Dither?"=w547:bool, "Offsets"=w543:T3, "Dither out"=w544:T43, "Message"=w541:string)  [unwired: 5 in, 1 out]
            n293 = case shown="True" w547 {
              tunnel: w543 -> [_ w570]
              tunnel: w553 -> [_ w569]
              tunnel: ["Next Step" "script Acquire Wait Move" ("Script State")] -> w551
              tunnel: ["Image acquisition and dithering complete." ("format string") w562] -> w546
              tunnel: w544 -> [_ w566]
              tunnel: w545 -> [w555 w564]
              tunnel: w541 -> [_ w562]
              frame False {
                w554 = 0.0 ("Value")
                n294 = call "CC Script Set Status Value.vi"("Value"=w554, "Ch Name"="Script Dither Total", "Data Q"=w555) -> ()  [unwired: 8 in, 1 out]
                n295 = call "CC Script Set Status Value.vi"("Value"=w554, "Ch Name"="Script Dither Count", "Data Q"=w555) -> ()  [unwired: 8 in, 1 out]
              }
              frame True {
                n296 = Unbundle By Name(w566) -> ("index"=w567:i32)
                n297 = Bundle By Name(cluster=T30 {"Cmd"="Offset", "Parameters"=variant} ("element"), "Parameters"=w570) -> (w572:T30)
                n298 = Increment(x=w567) -> (x+1=w565:i32)
                n299 = call "CC Script Set Status Value.vi"("Value"=w565, "Ch Name"="Script Dither Count", "Data Q"=w564) -> ()  [unwired: 8 in, 1 out]
                n300 = Enqueue Element(queue=w569, element=w572) -> (error out=w561:errorcluster)  [unwired: 2 in, 2 out]
                n301 = call "Stall Data Flow.vim"("value in"=w561, "milliseconds to wait"=u32 4000) -> ()  [unwired: 2 out]
              }
            }
            n302 = Unbundle By Name(w540) -> ("RA and DEC"=w542:T11)
            n303 = Get Date/Time In Seconds() -> (seconds since 1Jan1904=w549:timestamp)
            n304 = Bundle By Name(cluster=w552, "timer"=w549, "Target RA and DEC"=w542, "Dither"=w544, "Script State"=w551) -> (w550:T28)
            n305 = call "CC System Message.vi"("Message"=w546) -> ()  [unwired: 10 in, 1 out]
          }
          frame "script Telescope Move" {
            # "give telescope time to start\nmoving."
            n306 = Unbundle By Name(w576) -> ("Run Script"=w585:T5[], "step"=w584:i32, "Cmd Qs.Telescope Q"=w582:T2)
            n307 = Index Array(array=w585, index=w584) -> (element=w583:T5)
            n308 = Unbundle By Name(w583) -> ("Data"=w580:variant)
            n309 = Bundle By Name(cluster=T30 {"Cmd"="Move Focus", "Parameters"=variant} ("element"), "Parameters"=w580) -> (w579:T30)
            n310 = Enqueue Element(queue=w582, element=w579) -> (error out=w575:errorcluster)  [unwired: 2 in, 2 out]
            n311 = call "CC System Message.vi"("Message"="Script commanding telescope to move." ("format string")) -> ()  [unwired: 10 in, 1 out]
            n312 = call "Stall Data Flow.vim"("value in"=w575, "milliseconds to wait"=u32 2000) -> ()  [unwired: 2 out]
            n313 = Bundle By Name(cluster=w576, "Script State"="script Wait for Telescope Move") -> (w577:T28)
          }
          frame "script Telescope Home" {
            # "give telescope time to start\nmoving."
            n314 = Unbundle By Name(w589) -> ("Run Script"=w598:T5[], "step"=w597:i32, "Cmd Qs.Telescope Q"=w595:T2)
            n315 = Index Array(array=w598, index=w597) -> (element=w596:T5)
            n316 = Unbundle By Name(w596) -> ("Data"=w593:variant)
            n317 = Bundle By Name(cluster=T30 {"Cmd"="Home Focus", "Parameters"=variant} ("element"), "Parameters"=w593) -> (w592:T30)
            n318 = call "CC System Message.vi"("Message"="Script commanding telescope to home the focus." ("format string")) -> ()  [unwired: 10 in, 1 out]
            n319 = Enqueue Element(queue=w595, element=w592) -> (error out=w588:errorcluster)  [unwired: 2 in, 2 out]
            n320 = call "Stall Data Flow.vim"("value in"=w588, "milliseconds to wait"=u32 2000) -> ()  [unwired: 2 out]
            n321 = Bundle By Name(cluster=w589, "Script State"="script Wait for Telescope Move") -> (w590:T28)
          }
          frame "script Telescope RA DEC" {
            (unwired) CC_enum_Script_Action."Telescope RA DEC" ("Action")
            # "give telescope time to start\nmoving."
            n322 = Unbundle By Name(w612) -> ("Run Script"=w619:T5[], "step"=w618:i32, "at slit?"=w602:bool, "Cmd Qs.Telescope Q"=w616:T2)
            n323 = Index Array(array=w619, index=w618) -> (element=w617:T5)
            n324 = Unbundle By Name(w617) -> ("Data"=w609:variant)
            n325 = Variant To Data(type=T11 {"RA"=0.0, "DEC"=0.0} ("RA and DEC"), Variant=w609) -> (data=w607:T11)  [unwired: 1 in, 1 out]
            n326 = Select(t=T30 {"Cmd"="Offset", "Parameters"=variant} ("element"), s=w602, f=T30 {"Cmd"="Move", "Parameters"=variant} ("element")) -> (s? t:f=w599:T30)
            n327 = Bundle By Name(cluster=w599, "Parameters"=w609) -> (w615:T30)
            n328 = call "CC Convert RA and DEC to HHMMSS.vi"("RA and DEC"=w607) -> ("DEC String"=w605:string, "RA String"=w604:string)  [unwired: 7 in, 2 out]
            n329 = Enqueue Element(queue=w616, element=w615) -> (error out=w611:errorcluster)  [unwired: 2 in, 2 out]
            n330 = Format Into String(format string="Script commanding telescope to move to RA %s, DEC %s.", w604, w605) -> (resulting string=w603:string)  [unwired: 2 in, 1 out]
            n331 = call "CC System Message.vi"("Message"=w603) -> ()  [unwired: 10 in, 1 out]
            n332 = call "Stall Data Flow.vim"("value in"=w611, "milliseconds to wait"=u32 2000) -> ()  [unwired: 2 out]
            n333 = Bundle By Name(cluster=w612, "Script State"="script Wait for Telescope Move") -> (w613:T28)
          }
          frame "script Wait for Telescope Move" {
            n334 = call "CC Log Object.vi"("Action"=CC_enum_Current_Values_Action."Get Current Values") -> ("HK Channel out"=w631:refnum<class "HK Table.lvclass">)  [unwired: 8 in, 2 out]
            n335 = Unbundle By Name(w626) -> ("obj name"=w625:string)
            n336 = for {
              tunnel: w631 -> [w639]
              tunnel: string[] ["Telescope RA", "Telescope DEC", "Telescope Moving?", "Telescope Status"] -> [w638] mode=indexing
              tunnel: [w637] -> w629 mode=indexing
              n337 = call-dynamic "HK Read Value.vi"("Channel Name"=w638, "HK Channel in"=w639) -> ("Value"=w637:dbl)  [unwired: 4 in, 5 out]
            }
            n338 = Equal?(x=w625, y="NULL") -> (x = y?=w622:bool)
            n339 = Index Array(array=w629) -> (element #3=w628:dbl)  [unwired: 4 in, 3 out]
            n340 = Not(x=w622) -> (.not. x?=w621:bool)
            n341 = Greater Than 0?(x=w628) -> (x > 0?=w623:bool)
            n342 = And(x=w621, y=w623) -> (x .and. y?=w620:bool)
            n343 = case shown="False" w620 {
              tunnel: w626 -> [w635 w636]
              tunnel: [w633 w636] -> w627
              frame False {
                n344 = Bundle By Name(cluster=w635, "Script State"="Next Step") -> (w633:T28)
              }
              frame True {
              }
            }
          }
          frame "script Outlet" {
            n345 = Unbundle By Name(w650) -> ("Cmd Qs.CryoCooler Q"=w647:T2, "Parameters"=w648:variant)
            n346 = Variant To Data(type=T40 {"Outlet Idx"=0, "State"=FALSE} ("outlet parm in"), Variant=w648) -> (data=w643:T40)  [unwired: 1 in, 1 out]
            n347 = Bundle By Name(cluster=T30 {"Cmd"="SetOutlet", "Parameters"=variant} ("element"), "Parameters"=w643) -> (w645:T30)
            n348 = Unbundle By Name(w643) -> ("Outlet Idx"=w642:i32, "State"=w641:bool)
            n349 = Enqueue Element(queue=w647, element=w645) -> ()  [unwired: 2 in, 3 out]
            n350 = Format Into String(format string="Script sending outlet command: outlet %d to state %d", w642, w641) -> (resulting string=w640:string)  [unwired: 2 in, 1 out]
            n351 = call "CC System Message.vi"("Message"=w640) -> ()  [unwired: 10 in, 1 out]
          }
          frame "Ask User", "script Ask User" {
            n352 = Unbundle By Name(w651) -> ("Parameters"=w654:variant)
            n353 = Variant To Data(type="", Variant=w654) -> (data=w657:string, error out=w656:errorcluster)  [unwired: 1 in]
            n354 = case shown="No Error" w656 {
              tunnel: ["User Notification" ("Message") w660] -> w655
              tunnel: w654 -> [_ w662]
              frame No Error {
              }
              frame Error {
                n355 = call <vilib>:"Get Type Information.vi"("variant"=w662) -> ("name"=w661:string)  [unwired: 6 in, 4 out]
                n356 = Format Into String(format string="Software System Error in scripting. Ask User state parameter should be string but was not. Variant contents: %s", w661) -> (resulting string=w660:string)  [unwired: 2 in, 1 out]
              }
            }
            n357 = One Button Dialog(message=w657) -> ()  [unwired: 1 in, 1 out]
            n358 = Bundle By Name(cluster=w651, "Script State"="next step") -> (w652:T28)
            n359 = call "CC System Message.vi"("Message"=w655) -> ()  [unwired: 10 in, 1 out]
          }
          frame "script CmdLine" {
            n360 = Unbundle By Name(w666) -> ("Parameters"=w669:variant)
            n361 = Variant To Data(type="", Variant=w669) -> (data=w665:string, error out=w671:errorcluster)  [unwired: 1 in]
            n362 = case shown="No Error" w671 {
              tunnel: [w684 w686] -> w670
              tunnel: w669 -> [_ w688]
              tunnel: w665 -> [w679 _]
              tunnel: "Sending command to shell \"%s\"" ("Message") -> [w683 _]
              frame No Error {
                n363 = Concatenate Strings(w679, "\r\n") -> (w677:string)
                n364 = Format Into String(format string=w683, w679) -> (resulting string=w681:string, error out=w682:errorcluster)  [unwired: 2 in]
                n365 = call "CC System Message.vi"("error in (no error)"=w682, "Message"=w681) -> ("error out"=w680:errorcluster)  [unwired: 9 in]
                n366 = call <vilib>:"System Exec.vi"("error in (no error)"=w680, "standard input"=w677, "command line"="cmd") -> ("return code"=w674:i32, "standard error"=w673:string, "standard output"=w675:string)  [unwired: 5 in, 1 out]
                n367 = Format Into String(format string="Return Code: %d\nCommand stdout: %s\nCommand stderr: %s" ("Message"), w674, w675, w673) -> (resulting string=w684:string)  [unwired: 2 in, 1 out]
              }
              frame Error {
                n368 = call <vilib>:"Get Type Information.vi"("variant"=w688) -> ("name"=w687:string)  [unwired: 6 in, 4 out]
                n369 = Format Into String(format string="Software System Error in scripting. CmdLine parameter should be string but was not. Variant contents: %s", w687) -> (resulting string=w686:string)  [unwired: 2 in, 1 out]
              }
            }
            n370 = call "CC System Message.vi"("Message"=w670) -> ()  [unwired: 10 in, 1 out]
            n371 = Bundle By Name(cluster=w666, "Script State"="next step") -> (w667:T28)
          }
          frame "next step" {
            n372 = Unbundle By Name(w693) -> ("step"=w697:i32, "Run Script"=w696:T5[], "paused"=w690:bool)
            n373 = Increment(x=w697) -> (x+1=w692:i32)
            n374 = Array Size(array=w696) -> (size(s)=w695:i32)
            n375 = Greater Or Equal?(x=w692, y=w695) -> (x >= y?=w694:bool)
            n376 = case shown="False" w694 {
              tunnel: w693 -> [w701 w707]
              tunnel: w692 -> [w700 _]
              tunnel: [w699 w708] -> w691
              tunnel: w690 -> [w698 _]
              frame False {
                n377 = case shown="False" w698 {
                  tunnel: w701 -> [w705 w706]
                  tunnel: w700 -> [w704 _]
                  tunnel: [w703 w706] -> w699
                  frame False {
                    n378 = Bundle By Name(cluster=w705, "step"=w704, "Script State"="execute step" ("event data")) -> (w703:T28)
                  }
                  frame True {
                  }
                }
              }
              frame True {
                n379 = Bundle By Name(cluster=w707, "Script State"="end script" ("event data")) -> (w708:T28)
              }
            }
          }
          frame "end script" {
            w713 = "" ("Step Name")
            n380 = Unbundle By Name(w721) -> ("Script Settings.Script Name"=w724:string, "Script Status Q"=w719:refnum<queue>, "Data Q"=w710:refnum<queue>)
            n381 = Get Date/Time In Seconds() -> (seconds since 1Jan1904=w712:timestamp)
            n382 = Format Into String(format string="Script %s finished", w724) -> (resulting string=w725:string)  [unwired: 2 in, 1 out]
            n383 = call "CC Script Send Script End Status.vi"("Data Q"=w710) -> ()  [unwired: 10 in, 1 out]
            n384 = Bundle By Name(cluster=T35 {"Time"=timestamp(0 s since 1904-01-01), "Running"=FALSE, "Step"=0, "Script Name"="", "Step Name"=""}, "Running"=FALSE, "Step"=0, "Step Name"=w713, "Script Name"=w713, "Time"=w712) -> (w711:T35)
            n385 = call "CC System Message.vi"("Message"=w725) -> ()  [unwired: 10 in, 1 out]
            n386 = Bundle By Name(cluster=w721, "Script Running"=FALSE, "Script State"="idle") -> (w722:T28)
            n387 = Bundle By Name(cluster=T32 {"Msg"="Status", "Data"=variant} ("element"), "Data"=w711) -> (w717:T32)
            n388 = Enqueue Element(queue=w719, element=w717) -> ()  [unwired: 2 in, 3 out]
          }
          frame "abort script" {
            n389 = Unbundle By Name(w729) -> ("Script Settings.Script Name"=w731:string, "Script Running"=w728:bool)
            n390 = case shown="True" w728 {
              tunnel: w731 -> [_ w738]
              tunnel: [w733 w737] -> w730
              tunnel: w729 -> [w733 w736]
              tunnel: ["Script Abort received but script not running" w734] -> w727
              frame False {
              }
              frame True {
                n391 = Format Into String(format string="Script %s aborted.", w738) -> (resulting string=w734:string)  [unwired: 2 in, 1 out]
                n392 = Bundle By Name(cluster=w736, "Script State"="end script") -> (w737:T28)
              }
            }
            n393 = call "CC System Message.vi"("Message"=w727) -> ()  [unwired: 10 in, 1 out]
          }
          frame "script error" {
            n394 = Unbundle By Name(w740) -> ("Data Q"=w743:refnum<queue>)
            n395 = call "CC Script Set Status Value.vi"("Value"=2.0, "Ch Name"="Script State", "Data Q"=w743) -> ()  [unwired: 8 in, 1 out]
            n396 = Bundle By Name(cluster=w740, "Script State"="abort script") -> (w744:T28)
          }
          frame "Shutdown" {
            n397 = Unbundle By Name(w748) -> ("Script Settings"=w747:T4)
            n398 = call "Rd Wr Script Defaults.vi"("Write? (F:Read)"=TRUE, "Script Settings"=w747) -> ()  [unwired: 8 in, 2 out]
          }
        }
      }
      event "Script Path": Value Change {
        n399 = event-data() -> ()  [unwired: 1 in, 6 out]
        n400 = Unbundle By Name(w755) -> ("state"=w754:refnum<user-event>)
        n401 = Generate User Event(user event=w754, event data cluster="init" ("event data")) -> ()  [unwired: 2 in, 2 out]
        n402 = Bundle By Name(cluster=w755, "Script Settings.Script Path"="Script Path") -> (w752:T28)
        n403 = Unbundle By Name(w752) -> ("Script Settings"=w751:T4)
        n404 = call "Rd Wr Script Defaults.vi"("Write? (F:Read)"=TRUE, "Script Settings"=w751) -> ()  [unwired: 8 in, 2 out]
      }
      event "Script": Shortcut Menu Activation? {
        n405 = event-data() -> ("CtlRef"=w765:refnum<vi>, "MenuRef"=w763:refnum<k9>, "Coords"=w764:T44)  [unwired: 1 in, 1 out]
        n406 = Unbundle By Name(w758) -> ("Script Settings.Script Path"=w757:path)
        n407 = call "CC Rd Wr Script.vi"("Script Path"=w757, "Action"=CC_Rd_Wr_Script_Action."List") -> ("Script List"=w760:string[])  [unwired: 4 in, 5 out]
        n408 = invoke class="MCListbox (strict)" method="Point To Row Column"(reference=w765, "Point"=w764) -> ()  [unwired: 5 in, 7 out]
        n409 = for {
          tunnel: w760 -> [w768] mode=indexing
          tunnel: [w767] -> w759 mode=indexing
          n410 = Format Into String(format string="Insert|%s", w768) -> (resulting string=w767:string)  [unwired: 2 in, 1 out]
        }
        n411 = Insert Menu Items(5:"Insert" ("menu tag"), 7:w759, 8:w760, 9:w763) -> ()  [unwired: 2 in, 3 out]
        n412 = event-data("Discard?"=FALSE) -> ()  [unwired: 1 in, 1 out]
      }
      event "Script": Shortcut Menu Selection (User) {
        n413 = event-data() -> ("ItemTag"=w777:string, "CtlRef"=w782:refnum<vi>, "Coords"=w781:T44)  [unwired: 1 in, 5 out]
        n414 = Unbundle By Name(w773) -> ("state"=w771:refnum<user-event>, "Script"=w778:T5[], "Script Settings.Script Path"=w770:path)
        n415 = invoke class="MCListbox (strict)" method="Point To Row Column"(reference=w782, "Point"=w781) -> ("CellPosition"=w780:T45)  [unwired: 5 in, 6 out]
        n416 = Match Pattern(string=w777, regular expression="|") -> (before substring=w775:string, after substring=w774:string)  [unwired: 1 in, 2 out]
        n417 = Unbundle By Name(w780) -> ("Row"=w779:i32)
        n418 = case shown="\"Insert\"" w775 {
          tunnel: w779 -> [_ w786 w788 w807]
          tunnel: w778 -> [_ w787 _ w808]
          tunnel: w774 -> [_ _ _ w811]
          tunnel: w773 -> [w783 w784 w789 w802]
          tunnel: [w783 w784 w793 w800] -> w772
          tunnel: w771 -> [_ _ _ w799]
          tunnel: w770 -> [_ _ _ w796]
          frame "False", Default {
          }
          frame "Execute Step" {
            n419 = Index Array(array=w787, index=w786) -> (element=w785:T5)
            n420 = call "CC Script Execute Step.vi"("Script Step"=w785) -> ()  [unwired: 10 in, 1 out]
          }
          frame "Continue From This Step" {
            n421 = Unbundle By Name(w789) -> ("Script Settings.Script Name"=w791:string)
            n422 = Bundle By Name(cluster=w789, "step"=w788, "Script Running"=TRUE, "Script State"="execute step" ("event data")) -> (w793:T28)
            n423 = Format Into String(format string="Continuing Script \"%s\" from step %d" ("Message"), w791, w788) -> (resulting string=w790:string)  [unwired: 2 in, 1 out]
            n424 = call "CC System Message.vi"("Message"=w790) -> ()  [unwired: 10 in, 1 out]
          }
          frame "Insert" {
            n425 = Bundle By Name(cluster=T33 {"Name"="", "Script"=[]} ("Script"), "Name"=w811) -> (w810:T33)
            n426 = Increment(x=w807) -> (x+1=w797:i32)
            n427 = Generate User Event(user event=w799, event data cluster="show script" ("event data")) -> ()  [unwired: 2 in, 2 out]
            n428 = Split 1D Array(array=w808, index=w797) -> (first subarray=w804:T5[], second subarray=w805:T5[])
            n429 = call "CC Rd Wr Script.vi"("Script Path"=w796, "Action"=CC_Rd_Wr_Script_Action."Read", "Script"=w810) -> ("Script"=w806:T33)  [unwired: 3 in, 5 out]
            n430 = Unbundle By Name(w806) -> ("Script"=w803:T5[])
            n431 = Build Array (concatenate)(w804, w803, w805) -> (w801:T5[])
            n432 = Bundle By Name(cluster=w802, "Script"=w801) -> (w800:T28)
          }
        }
      }
      event "Script": Value Change {
        n433 = event-data() -> ("NewVal"=w817:string)  [unwired: 1 in]
        n434 = Unbundle By Name(w815) -> ("state"=w814:refnum<user-event>)
        n435 = Generate User Event(user event=w814, event data cluster="load script" ("event data")) -> ()  [unwired: 2 in, 2 out]
        n436 = Bundle By Name(cluster=w815, "Script Settings.Script Name"=w817) -> (w816:T28)
      }
      event "Edit Script", "New Script": Value Change {
        n437 = event-data() -> ()  [unwired: 1 in, 6 out]
        n438 = Unbundle By Name(w820) -> ("script edit ref"=w819:refnum<vi>)
        n439 = property class="VI Interface Type 0"(reference=w819) -> ("FP.State"=w818:T46)  [unwired: 1 in, 2 out]
        n440 = Select(t="", s="New Script", f="Script") -> (s? t:f=w822:string)
        n441 = case shown="\"Invalid\", Default" w818 {
          tunnel: w822 -> [w830 _]
          tunnel: [w829 w837] -> w821
          tunnel: w820 -> [w828 w837]
          tunnel: w819 -> [_ w839]
          frame "Invalid", Default {
            n442 = vi-ref "CC Create Script.vi"() -> (w835:refnum<vi>)
            n443 = property class="VI (strict)"(reference=w835) -> (error out=w836:errorcluster, "Path"=w834:path)  [unwired: 1 in, 1 out]
            n444 = Open VI Reference(type specifier VI Refnum (for type only)=w835, vi path=w834, options=128, error in (no error)=w836) -> (vi reference=w833:refnum<vi>, error out=w831:errorcluster)  [unwired: 2 in]
            n445 = call-by-ref "Start Asynchronous Call"(reference=w833, error in=w831, "script name in"=w830) -> (reference out=w827:refnum<vi>)  [unwired: 10 in, 2 out]
            n446 = invoke class="VI Interface Type 0" method="FP.Open"(reference=w827, "Activate"=TRUE ("Activate?")) -> ()  [unwired: 3 in, 5 out]
            n447 = Bundle By Name(cluster=w828, "script edit ref"=w827) -> (w829:T28)
          }
          frame "Standard" {
            n448 = property class="VI Interface Type 0"(reference=w839, "Front Panel.IsFrontmost"=TRUE ("Front Panel Window:Is Frontmost")) -> ()  [unwired: 1 in, 2 out]
          }
        }
      }
      event "Run Script": Value Change {
        n449 = event-data() -> ()  [unwired: 1 in, 6 out]
        n450 = Unbundle By Name(w842) -> ("state"=w841:refnum<user-event>)
        n451 = Generate User Event(user event=w841, event data cluster="start script" ("event data")) -> ()  [unwired: 2 in, 2 out]
      }
      event "Stop Script": Value Change {
        n452 = event-data() -> ()  [unwired: 1 in, 6 out]
        n453 = Unbundle By Name(w845) -> ("state"=w844:refnum<user-event>)
        n454 = Generate User Event(user event=w844, event data cluster="abort script" ("event data")) -> ()  [unwired: 2 in, 2 out]
      }
      event "Close": Value Change {
        n455 = event-data() -> ()  [unwired: 1 in, 2 out]
        n456 = Unbundle By Name(w848) -> ("state"=w847:refnum<user-event>)
        n457 = Generate User Event(user event=w847, event data cluster="shutdown" ("event data")) -> ()  [unwired: 2 in, 2 out]
      }
    }
  }
